vi "GFITS_API.vi"(0 "modpath":path, 7 "Cmd":string, 11 "error in":errorcluster) -> (4 "ImmedReplyString":string, 15 "error out":errorcluster)   [LabVIEW 2016]
uses:
  DBSHAND/private/vis/DatabaseHand_Element_Set(string).vi
  DBSHAND/private/vis/DatabaseHand_Element_Set(bool).vi
  DBSHAND/private/vis/DatabaseHand_Element_Get(U32).vi
  DBSHAND/private/vis/DatabaseHand_Element_Get(string).vi
  DBSHAND/private/vis/DatabaseHand_Element_Get(bool).vi
  DBSHAND/private/vis/DatabaseHand_Element_Get(I32).vi
  private/vis/GFITS_Gbls.vi
panel:
  out "origautonum":bool
  in  "cmd struct":T1
  out "auxhdr":path
  out "caller path":path
  in  "Module vi name":string="GFITS_Main.vi"
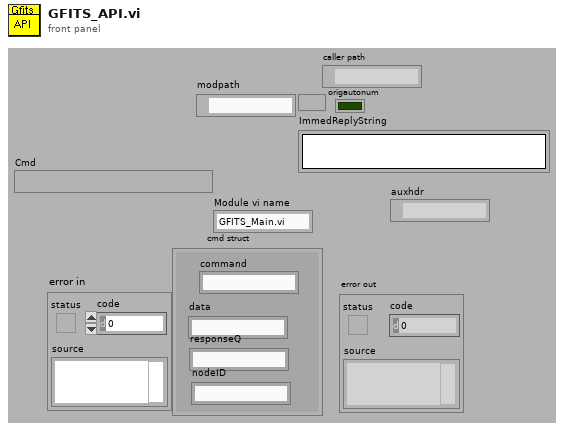
[diagram p1: front panel]
types:
  T1 = cluster{"command":string, "data":string, "responseQ":string, "nodeID":string}
  T2 = typedef "DatabaseHand_RefNum.ctl" = refnum<vi>
  T3 = cluster{"name":string, "Path":path, "bitpix":i8, "naxis":u8, "naxes":u32[], "datatype":u16, "multiple extensions":bool, "hdutype":u16, "writeToDisk":bool, "num_of_ext":u8, "file ref":i32, "createnewimage":bool}
  T4 = cluster{"Name":string, "size (bytes)":u32, "pointer":u32, "Lock":bool}
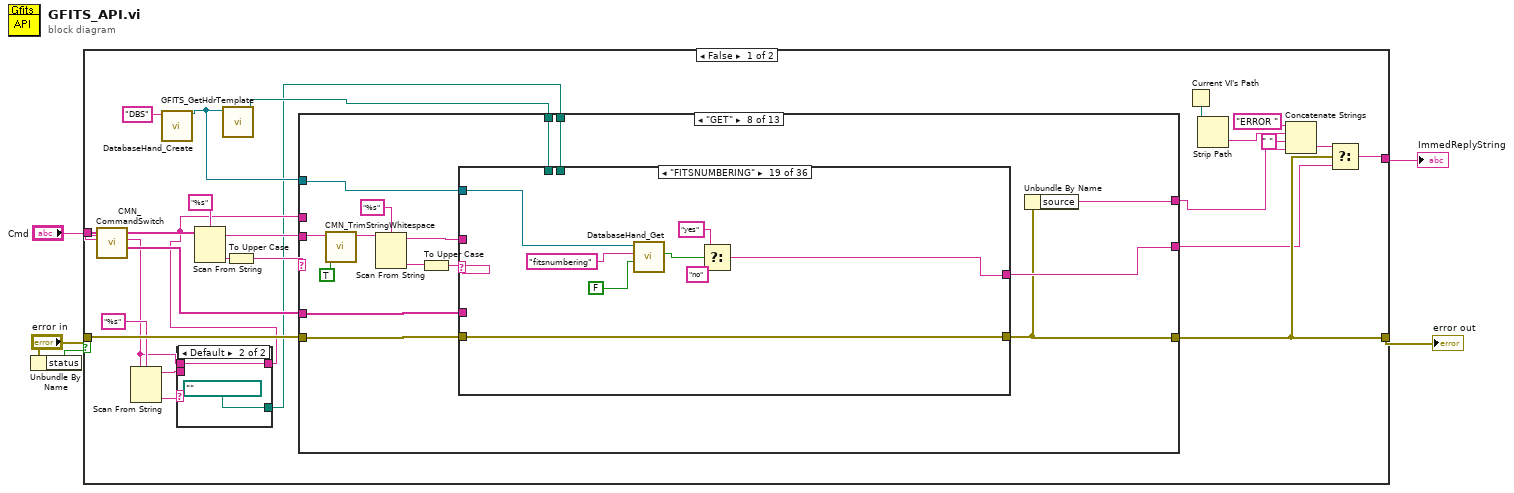
[diagram p0: block diagram]
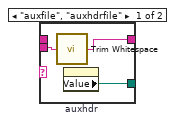
[diagram p2: hidden frame]
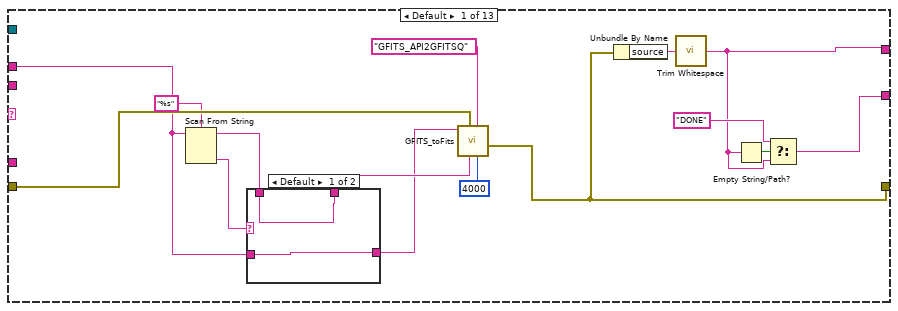
[diagram p3: hidden frame]
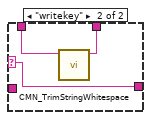
[diagram p4: hidden frame]
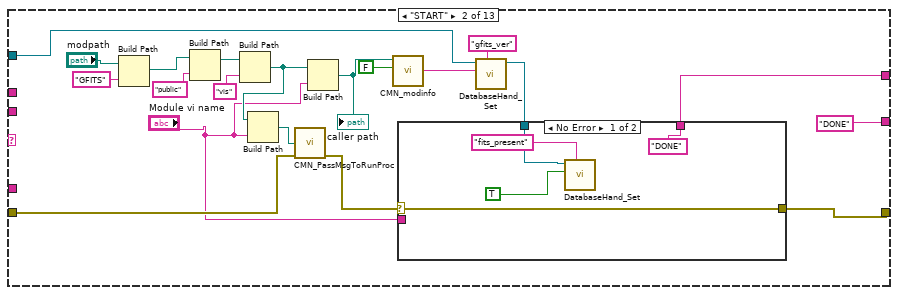
[diagram p5: hidden frame]
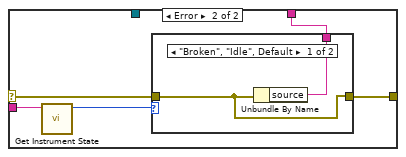
[diagram p6: hidden frame]
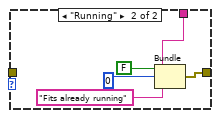
[diagram p7: hidden frame]
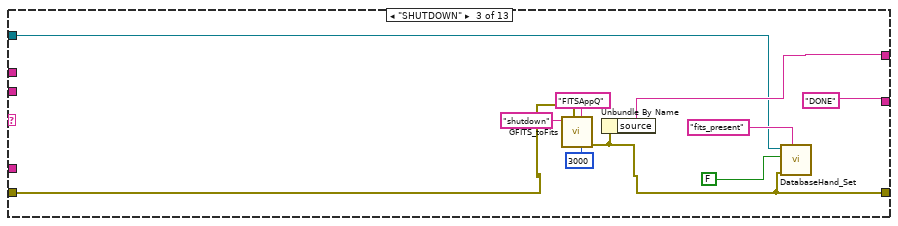
[diagram p8: hidden frame]
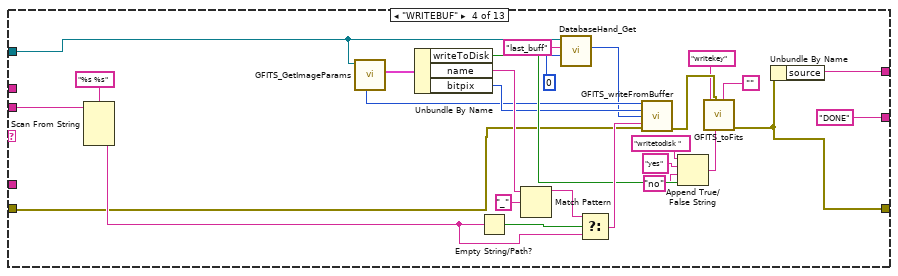
[diagram p9: hidden frame]
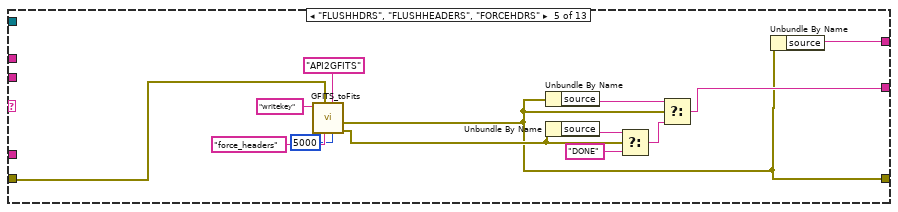
[diagram p10: hidden frame]
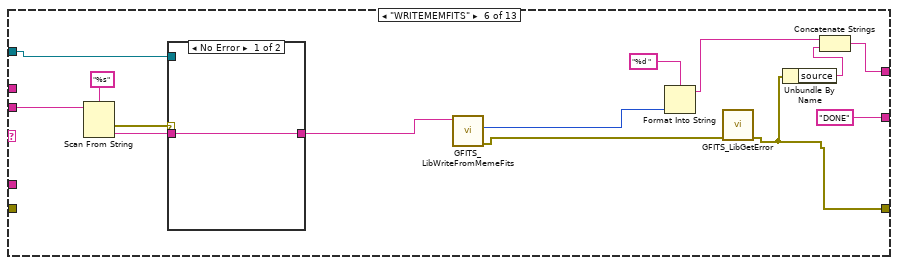
[diagram p11: hidden frame]
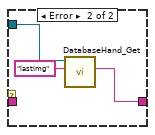
[diagram p12: hidden frame]
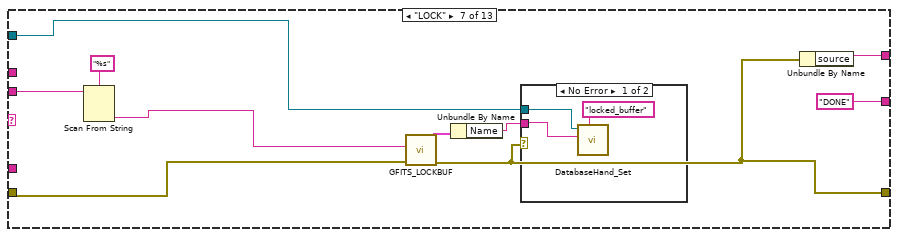
[diagram p13: hidden frame]
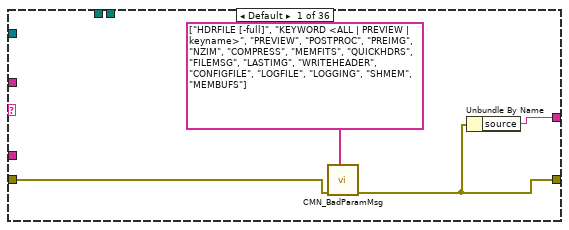
[diagram p15: hidden frame]
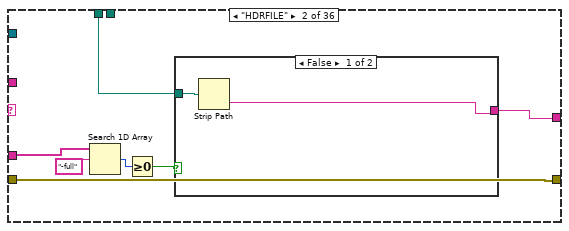
[diagram p16: hidden frame]
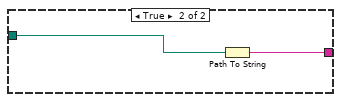
[diagram p17: hidden frame]
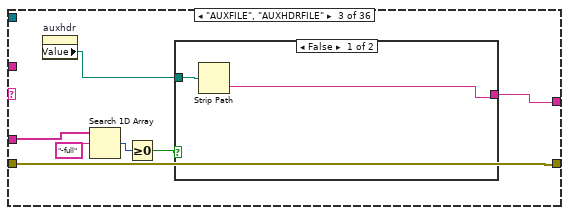
[diagram p18: hidden frame]
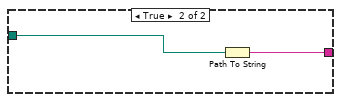
[diagram p19: hidden frame]
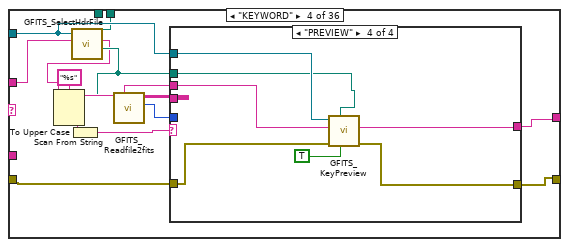
[diagram p20: hidden frame]
diagram:
  n1 = Unbundle By Name("error in") -> ("status"=w3:bool)
  n2 = case shown="False" w3 {
    tunnel: "error in" -> [w30 w1388]
    tunnel: [w23 w1388] -> w1
    tunnel: [w22 ""] -> w5
    tunnel: "Cmd" -> [w19 _]
    frame False {
      n3 = call "CMN_CommandSwitch.vi"("command in"=w19) -> ("swhitches"=w18:string[], "command out"=w9:string)  [unwired: 1 in, 8 out]
      n4 = Scan From String(format string="%s", input string=w9) -> (remaining string=w7:string, output 1=w10:string)  [unwired: 2 in, 3 out]
      n5 = call "DatabaseHand_Create.vi"("Name"="DBS") -> ("Database RefNum out"=w15:T2)  [unwired: 1 in, 9 out]
      n6 = case shown="Default" w10 {
        tunnel: w9 -> [_ w35]
        tunnel: [w32 w35] -> w8
        tunnel: w7 -> [w33 _]
        tunnel: [w31 path "" ("auxhdr")] -> w6
        frame "auxfile", "auxhdrfile" {
          n7 = call <vilib>:"Trim Whitespace.vi"("string"=w33) -> ("trimmed string"=w32:string)  [unwired: 1 in]
          n8 = property on="auxhdr" class="Path"() -> ("Value"=w31:path)  [unwired: 2 in, 2 out]
        }
        frame Default {
        }
      }
      n9 = Scan From String(format string="%s" ("Format String"), input string=w8) -> (remaining string=w20:string, output 1=w29:string)  [unwired: 2 in, 3 out]
      n10 = call "GFITS_GetHdrTemplate.vi"("Database RefNum"=w15) -> ("path"=w16:path)  [unwired: 10 out]
      n11 = To Upper Case(1:w29) -> (0:w14:string)
      n12 = case shown="\"GET\"" w14 {
        selector: w14 -> [_ _ _ _ _ _ _ _ _ _ _ _ w1386]
        tunnel: w30 -> [w49 w58 w100 w110 w129 _ w166 w180 w501 w1241 w1366 w1370 w1385]
        tunnel: [w48 w74 w93 w120 w130 w145 w163 w179 w500 w1240 w1365 w1370 w1384] -> w23
        tunnel: [w42 w61 w99 w125 w141 w142 w164 w185 w506 w1245 w1367 w1371 w1383] -> w13
        tunnel: [w41 "DONE" "DONE" "DONE" w131 "DONE" "DONE" w181 w502 w1242 w1367 w1371 w1383] -> w21
        tunnel: w20 -> [_ _ _ w128 _ w155 w169 w187 w508 w1247 _ w1369 _]
        tunnel: w18 -> [_ _ _ _ _ _ _ w178 w498 _ w1364 _ _]
        tunnel: w16 -> [_ _ _ _ _ _ _ w177 w497 w1236 _ _ _]
        tunnel: w15 -> [_ w62 w92 w102 _ w149 w160 w175 w496 w1238 _ _ _]
        tunnel: w8 -> [w36 _ _ _ _ _ _ _ _ _ _ _ _]
        tunnel: w6 -> [_ _ _ _ _ _ _ w173 w494 w1232 _ _ _]
        frame Default {
          n13 = Scan From String(format string="%s", input string=w36) -> (remaining string=w39:string, output 1=w40:string)  [unwired: 2 in, 3 out]
          n14 = case shown="Default" w40 {
            selector: w40 -> [_ w53]
            tunnel: w39 -> [w51 w55]
            tunnel: [w51 w54] -> w38
            tunnel: [w52 w53] -> w37
            tunnel: w36 -> [w52 _]
            frame Default {
            }
            frame "writekey" {
              n15 = call "CMN_TrimStringWhitespace.vi"("string"=w55) -> ("trimmed string"=w54:string)  [unwired: 1 in, 8 out]
            }
          }
          n16 = call "GFITS_toFits.vi"("ms timeout (-1)"=4000, "response Q"="GFITS_API2GFITSQ", "key"=w38, "error in (no error)"=w49, "command"=w37) -> ("response"=w48:errorcluster)  [unwired: 4 in, 2 out]
          n17 = Unbundle By Name(w48) -> ("source"=w47:string)
          n18 = call <vilib>:"Trim Whitespace.vi"("string"=w47) -> ("trimmed string"=w42:string)  [unwired: 1 in]
          n19 = Empty String/Path?(string/path=w42) -> (empty?=w44:bool)
          n20 = Select(t="DONE", s=w44, f=w42) -> (s? t:f=w41:string)
        }
        frame "START" {
          n21 = Build Path(base path="modpath", name or relative path="GFITS") -> (appended path=w69:path)
          n22 = Build Path(base path=w69, name or relative path="public") -> (appended path=w71:path)
          n23 = Build Path(base path=w71, name or relative path="vis") -> (appended path=w60:path)
          n24 = Build Path(base path=w60, name or relative path="Module vi name") -> (appended path=w59:path)
          n25 = call "CMN_PassMsgToRunProc.vi"("VItoRun"=w59, "error in (no error)"=w58) -> ("error out"=w75:errorcluster)  [unwired: 1 in, 12 out]
          n26 = Build Path(base path=w60, name or relative path="Module vi name") -> (appended path=w66:path)
          "caller path" <- w66
          n27 = call "CMN_modinfo.vi"("full"=FALSE, "caller path"=w66) -> ("INFO"=w63:string)  [unwired: 1 in, 8 out]
          n28 = call-poly "DatabaseHand_Set.vi"("name"="gfits_ver", "value"=w63, "Database RefNum in"=w62) -> ("Database RefNum out"=w56:T2)  [unwired: 5 in, 3 out]
          n29 = case shown="No Error" w75 {
            selector: w75 -> [w80 w85]
            tunnel: [w80 w81] -> w74
            tunnel: ["DONE" ("source") w84] -> w61
            tunnel: "Module vi name" -> [_ w83]
            tunnel: w56 -> [w78 _]
            frame No Error {
              n30 = call-poly "DatabaseHand_Set.vi"("name"="fits_present", "value"=TRUE ("full"), "Database RefNum in"=w78) -> ()  [unwired: 5 in, 4 out]
            }
            frame Error {
              n31 = call <vilib>:"Get Instrument State.vi"("VI name"=w83) -> ("vi state"=w82:enum32{"Broken", "Idle", "Running"})  [unwired: 1 in, 9 out]
              n32 = case shown="\"Broken\", \"Idle\", Default" w82 {
                tunnel: w85 -> [w86 _]
                tunnel: [w87 w88] -> w84
                tunnel: [w86 w91] -> w81
                frame "Broken", "Idle", Default {
                  n33 = Unbundle By Name(w86) -> ("source"=w87:string)
                }
                frame "Running" {
                  w88 = "Fits already running"
                  n34 = Bundle(FALSE, 0, w88) -> (w91:errorcluster)  [unwired: 1 out]
                }
              }
            }
          }
        }
        frame "SHUTDOWN" {
          n35 = call "GFITS_toFits.vi"("ms timeout (-1)"=3000, "response Q"="FITSAppQ", "error in (no error)"=w100, "command"="shutdown" ("Command")) -> ("error out"=w93:errorcluster)  [unwired: 5 in, 2 out]
          n36 = Unbundle By Name(w93) -> ("source"=w99:string)
          n37 = call-poly "DatabaseHand_Set.vi"("name"="fits_present", "error in (no error)"=w93, "value"=FALSE ("full"), "Database RefNum in"=w92) -> ()  [unwired: 4 in, 4 out]
        }
        frame "WRITEBUF" {
          n38 = Scan From String(format string="%s %s" ("Format String"), input string=w128) -> (output 2=w123:string)  [unwired: 2 in, 6 out]
          n39 = call "GFITS_GetImageParams.vi"("Database RefNum"=w102) -> ("imageStruct"=w107:T3, "totele"=w106:u32)  [unwired: 1 in, 8 out]
          n40 = Unbundle By Name(w107) -> ("writeToDisk"=w118:bool, "name"=w113:string, "bitpix"=w109:i8)
          n41 = Empty String/Path?(string/path=w123) -> (empty?=w124:bool)
          n42 = Match Pattern(string=w113, regular expression="_") -> (before substring=w111:string)  [unwired: 4 out]
          n43 = call-poly "DatabaseHand_Get.vi"("default value"=u32 0 ("last_buff"), "name"="last_buff", "Database RefNum in"=w102) -> ("value"=w103:u32)  [unwired: 2 in, 6 out]
          n44 = Select(t=w111, s=w124, f=w123) -> (s? t:f=w122:string)
          n45 = call "GFITS_writeFromBuffer.vi"("total pixels"=w106, "bpp"=w109, "buffer pointer"=w103, "name"=w122, "error in (no error)"=w110) -> ("error out"=w121:errorcluster)  [unwired: 2 in, 8 out]
          n46 = Append True/False String(1:w118, 2:"no" ("false string"), 3:"yes" ("true string"), 4:"writetodisk " ("string (\"\")")) -> (0:w114:string)
          n47 = call "GFITS_toFits.vi"("response Q"="", "key"=w114, "error in (no error)"=w121, "command"="writekey") -> ("error out"=w120:errorcluster)  [unwired: 5 in, 2 out]
          n48 = Unbundle By Name(w120) -> ("source"=w125:string)
        }
        frame "FLUSHHDRS", "FLUSHHEADERS", "FORCEHDRS" {
          n49 = call "GFITS_toFits.vi"("ms timeout (-1)"=5000, "response Q"="API2GFITS", "key"="force_headers", "error in (no error)"=w129, "command"="writekey") -> ("error out"=w132:errorcluster, "response"=w130:errorcluster)  [unwired: 4 in, 1 out]
          n50 = Unbundle By Name(w130) -> ("source"=w136:string)
          n51 = Unbundle By Name(w132) -> ("source"=w135:string)
          n52 = Select(t=w135, s=w132, f="DONE") -> (s? t:f=w134:string)
          n53 = Select(t=w136, s=w130, f=w134) -> (s? t:f=w131:string)
          n54 = Unbundle By Name(w130) -> ("source"=w141:string)
        }
        frame "WRITEMEMFITS" {
          n55 = Scan From String(format string="%s" ("Format String"), input string=w155) -> (error out=w152:errorcluster, output 1=w151:string)  [unwired: 2 in, 3 out]
          n56 = case shown="No Error" w152 {
            tunnel: w151 -> [w156 _]
            tunnel: [w156 w157] -> w150
            tunnel: w149 -> [_ w159]
            frame No Error {
            }
            frame Error {
              n57 = call-poly "DatabaseHand_Get.vi"("name"="lastimg", "Database RefNum in"=w159) -> ("value"=w157:string)  [unwired: 3 in, 6 out]
            }
          }
          n58 = call "GFITS_LibWriteFromMemeFits.vi"("imname"=w150) -> ("error out"=w146:errorcluster, "return value"=w148:i32)  [unwired: 1 in, 8 out]
          n59 = Format Into String(format string="%d ", w148) -> (resulting string=w144:string)  [unwired: 2 in, 1 out]
          n60 = call "GFITS_LibGetError.vi"("error in (no error)"=w146) -> ("error out"=w145:errorcluster)  [unwired: 10 out]
          n61 = Unbundle By Name(w145) -> ("source"=w143:string)
          n62 = Concatenate Strings(w144, w143) -> (w142:string)
        }
        frame "LOCK" {
          n63 = Scan From String(format string="%s" ("Format String"), input string=w169) -> (output 1=w165:string)  [unwired: 2 in, 4 out]
          n64 = call "GFITS_LOCKBUF.vi"("error in"=w166, "bufname"=w165) -> ("error out"=w163:errorcluster, "locked buffer"=w162:T4)  [unwired: 8 out]
          n65 = Unbundle By Name(w162) -> ("Name"=w161:string)
          n66 = case shown="No Error" w163 {
            tunnel: w161 -> [w170 _]
            tunnel: w160 -> [w172 _]
            frame No Error {
              n67 = call-poly "DatabaseHand_Set.vi"("name"="locked_buffer", "value"=w170, "Database RefNum in"=w172) -> ()  [unwired: 5 in, 4 out]
            }
            frame Error {
            }
          }
          n68 = Unbundle By Name(w163) -> ("source"=w164:string)
        }
        frame "GET" {
          n69 = call "CMN_TrimStringWhitespace.vi"("Both Ends?(T)"=TRUE, "string"=w187) -> ("trimmed string"=w184:string)  [unwired: 8 out]
          n70 = Scan From String(format string="%s" ("Format String"), input string=w184) -> (remaining string=w176:string, output 1=w183:string)  [unwired: 2 in, 3 out]
          n71 = To Upper Case(1:w183) -> (0:w174:string)
          n72 = case shown="\"FITSNUMBERING\"" w174 {
            tunnel: [w188 w198 w209 w221 w265 w268 w273 w279 w285 w292 w299 w307 w315 w323 w331 w339 w345 w349 w357 w368 w376 w384 w389 w398 w405 w412 w419 w426 w433 w438 w448 w450 w463 w471 w477 w480] -> w181
            tunnel: w180 -> [w190 w197 w208 w222 w267 w271 w276 w282 w288 w295 w302 w310 w318 w326 w334 w342 w344 w355 w363 w371 w379 w387 w395 w401 w408 w415 w422 w429 w436 w440 w445 w456 w467 w473 w479 w487]
            tunnel: [w189 w197 w208 w220 w266 w271 w275 w281 w287 w294 w301 w309 w317 w325 w333 w341 w344 w355 w363 w370 w378 w386 w395 w400 w407 w414 w421 w428 w435 w439 w445 w456 w467 w473 w479 w486] -> w179
            tunnel: w178 -> [_ w196 w207 _ _ _ _ _ _ _ _ _ _ _ _ _ _ _ _ _ _ _ _ _ _ _ _ _ _ _ _ _ _ _ _ _]
            tunnel: w177 -> [_ w192 _ _ _ _ _ _ _ _ _ _ _ _ _ _ _ _ _ _ _ _ _ _ _ _ _ _ _ _ _ _ _ _ _ _]
            tunnel: w176 -> [_ _ _ w214 w263 w269 _ _ _ _ _ _ _ _ _ _ _ _ _ _ _ _ _ _ _ _ _ _ _ _ _ w451 _ _ _ _]
            tunnel: w175 -> [_ _ _ w218 w264 w270 _ _ _ _ _ _ _ _ _ _ w348 w356 w364 _ _ _ w394 _ _ _ _ _ _ _ w449 w455 _ _ _ _]
            tunnel: w173 -> [_ _ _ w217 w260 _ _ _ _ _ _ _ _ _ _ _ _ _ _ _ _ _ _ _ _ _ _ _ _ _ _ _ _ _ _ _]
            frame Default {
              n73 = call "CMN_BadParamMsg.vi"("valid params"=string[] ["HDRFILE [-full]", "KEYWORD <ALL | PREVIEW | keyname>", "PREVIEW", "POSTPROC", "PREIMG", "NZIM", "COMPRESS", "MEMFITS", "QUICKHDRS", "FILEMSG", "LASTIMG", "WRITEHEADER", "CONFIGFILE", "LOGFILE", "LOGGING", "SHMEM", "MEMBUFS"], "error in (no error)"=w190) -> ("error out"=w189:errorcluster)  [unwired: 2 in, 7 out]
              n74 = Unbundle By Name(w189) -> ("source"=w188:string)
            }
            frame "HDRFILE" {
              n75 = Search 1D Array(1D array=w196, element="-full") -> (index of element=w194:i32)  [unwired: 1 out]
              n76 = Greater Or Equal To 0?(x=w194) -> (x >= 0?=w193:bool)
              n77 = case shown="False" w193 {
                tunnel: [w199 w202] -> w198
                tunnel: w192 -> [w200 w201]
                frame False {
                  n78 = Strip Path(path=w200) -> (name=w199:string)  [unwired: 1 out]
                }
                frame True {
                  n79 = Path To String(path=w201) -> (string=w202:string)
                }
              }
            }
            frame "AUXFILE", "AUXHDRFILE" {
              n80 = property on="auxhdr" class="Path"() -> ("Value"=w203:path)  [unwired: 2 in, 2 out]
              n81 = Search 1D Array(1D array=w207, element="-full") -> (index of element=w205:i32)  [unwired: 1 out]
              n82 = Greater Or Equal To 0?(x=w205) -> (x >= 0?=w204:bool)
              n83 = case shown="False" w204 {
                tunnel: [w210 w213] -> w209
                tunnel: w203 -> [w211 w212]
                frame False {
                  n84 = Strip Path(path=w211) -> (name=w210:string)  [unwired: 1 out]
                }
                frame True {
                  n85 = Path To String(path=w212) -> (string=w213:string)
                }
              }
            }
            frame "KEYWORD" {
              n86 = call "GFITS_SelectHdrFile.vi"("auxhdr"=w217, "line in"=w214, "Database RefNum"=w218) -> ("path out"=w216:path, "line out"=w215:string)  [unwired: 7 out]
              n87 = Scan From String(format string="%s" ("Format String"), input string=w215) -> (remaining string=w219:string, output 1=w224:string)  [unwired: 2 in, 3 out]
              n88 = To Upper Case(1:w224) -> (0:w223:string)
              n89 = call "GFITS_Readfile2fits.vi"("file"=w216) -> ("number of after keywords"=w225:i32, "after Keywords"=w226:string[][])  [unwired: 1 in, 8 out]
              n90 = case shown="\"PREVIEW\"" w223 {
                selector: w223 -> [_ w240 _ _]
                tunnel: w226 -> [_ w242 w250 _]
                tunnel: w216 -> [_ _ w249 w253]
                tunnel: w225 -> [_ _ _ _]
                tunnel: [w229 w235 w246 w256] -> w221
                tunnel: w222 -> [w232 w233 w248 w258]
                tunnel: [w231 w233 w247 w257] -> w220
                tunnel: w218 -> [_ _ _ w255]
                tunnel: w219 -> [_ _ _ w254]
                frame "", " " {
                  w229 = " nothing to get"
                  n91 = Bundle By Name(cluster=w232, "source"=w229, "code"=-22, "status"=FALSE) -> (w231:errorcluster)
                }
                frame Default {
                  w239 = 0 ("Index")
                  n92 = Build Array(w242) -> (w241:string[][][])
                  n93 = call "GFITS_FindKeywordFromArray.vi"("Keyword"=w240, "Keywords"=w241) -> ("values"=w237:string[][], "indexes"=w238:i16[])  [unwired: 8 out]
                  n94 = Index Array(array=w238, index=w239) -> (element=w236:i16)
                  n95 = Index Array(array=w237, index (row)=w239) -> (element=w234:string[])  [unwired: 1 in]
                  n96 = case shown="Default" w236 {
                    tunnel: ["NOT FOUND" w244] -> w235
                    tunnel: w234 -> [_ w245]
                    frame -1 {
                    }
                    frame Default {
                      n97 = call "CMN_Arr2Str.vi"("Array in"=w245) -> ("string out"=w244:string)  [unwired: 10 out]
                    }
                  }
                }
                frame "ALL" {
                  n98 = call "GFITS_Fits2File.vi"("write to file?"=FALSE, "error in (no error)"=w248, "Keywords"=w250, "filename"=w249) -> ("error out"=w247:errorcluster, "string out"=w246:string)  [unwired: 1 in, 5 out]
                }
                frame "PREVIEW" {
                  n99 = call "GFITS_KeyPreview.vi"("nd queue"=TRUE, "template path"=w253, "error in (no error)"=w258, "args"=w254, "Database RefNum in"=w255) -> ("error out"=w257:errorcluster, "preview"=w256:string)  [unwired: 5 out]
                }
              }
            }
            frame "PREVIEW" {
              n100 = call "GFITS_SelectHdrFile.vi"("auxhdr"=w260, "line in"=w263, "Database RefNum"=w264) -> ("path out"=w261:path, "line out"=w262:string)  [unwired: 7 out]
              n101 = call "GFITS_KeyPreview.vi"("nd queue"=TRUE, "template path"=w261, "error in (no error)"=w267, "args"=w262, "Database RefNum in"=w264) -> ("error out"=w266:errorcluster, "preview"=w265:string)  [unwired: 5 out]
            }
            frame "GEOMPREVIEW", "GEOMUPDATE" {
              n102 = call "GFITS_GeomKeyPreview.vi"("args"=w269, "Database RefNum in"=w270) -> ("preview"=w268:string)  [unwired: 1 in, 8 out]
            }
            frame "CONFIGFILE" {
              n103 = call "GFITS_toFits.vi"("response Q"="API2GFITS", "error in (no error)"=w276, "command"="GET CONFIGFILE") -> ("error out"=w275:errorcluster, "response"=w274:errorcluster)  [unwired: 6 in, 1 out]
              n104 = Unbundle By Name(w274) -> ("source"=w273:string)
            }
            frame "LOGFILE" {
              n105 = call "GFITS_toFits.vi"("response Q"="API2GFITS", "error in (no error)"=w282, "command"="GET LOGFILE") -> ("error out"=w281:errorcluster, "response"=w280:errorcluster)  [unwired: 6 in, 1 out]
              n106 = Unbundle By Name(w280) -> ("source"=w279:string)
            }
            frame "LOGGING" {
              n107 = call "GFITS_toFits.vi"("response Q"="API2GFITS", "error in (no error)"=w288, "command"="GET LOGGING") -> ("error out"=w287:errorcluster, "response"=w286:errorcluster)  [unwired: 6 in, 1 out]
              n108 = Unbundle By Name(w286) -> ("source"=w285:string)
            }
            frame "MEMBUF" {
              n109 = call "GFITS_toFits.vi"("response Q"="API2GFITS", "key"="get_membufptr", "error in (no error)"=w295, "command"="writekey") -> ("error out"=w294:errorcluster, "response"=w293:errorcluster)  [unwired: 5 in, 1 out]
              n110 = Unbundle By Name(w293) -> ("source"=w292:string)
            }
            frame "EXTENSIONSMAP", "EXTMAP", "MAPEXTENSIONS" {
              n111 = call "GFITS_toFits.vi"("response Q"="API2GFITS", "key"="get_extensionsmap", "error in (no error)"=w302, "command"="writekey") -> ("error out"=w301:errorcluster, "response"=w300:errorcluster)  [unwired: 5 in, 1 out]
              n112 = Unbundle By Name(w300) -> ("source"=w299:string)
            }
            frame "MEMFITS" {
              n113 = call "GFITS_toFits.vi"("ms timeout (-1)"=5000, "response Q"="API2GFITS", "key"="get_memfits", "error in (no error)"=w310, "command"="writekey") -> ("error out"=w309:errorcluster, "response"=w308:errorcluster)  [unwired: 4 in, 1 out]
              n114 = Unbundle By Name(w308) -> ("source"=w307:string)
            }
            frame "MEMHDRS" {
              n115 = call "GFITS_toFits.vi"("ms timeout (-1)"=5000, "response Q"="API2GFITS", "key"="get_memhdrs", "error in (no error)"=w318, "command"="writekey") -> ("error out"=w317:errorcluster, "response"=w316:errorcluster)  [unwired: 4 in, 1 out]
              n116 = Unbundle By Name(w316) -> ("source"=w315:string)
            }
            frame "POSTPROC" {
              n117 = call "GFITS_toFits.vi"("ms timeout (-1)"=5000, "response Q"="API2GFITS", "key"="get_postproc", "error in (no error)"=w326, "command"="writekey") -> ("error out"=w325:errorcluster, "response"=w324:errorcluster)  [unwired: 4 in, 1 out]
              n118 = Unbundle By Name(w324) -> ("source"=w323:string)
            }
            frame "PREIMAGE", "PREIMAGESCRIPT", "PREIMG" {
              n119 = call "GFITS_toFits.vi"("ms timeout (-1)"=5000, "response Q"="API2GFITS", "key"="get_preimg", "error in (no error)"=w334, "command"="writekey") -> ("error out"=w333:errorcluster, "response"=w332:errorcluster)  [unwired: 4 in, 1 out]
              n120 = Unbundle By Name(w332) -> ("source"=w331:string)
            }
            frame "TESTDIR", "TMPDIR" {
              n121 = call "GFITS_toFits.vi"("ms timeout (-1)"=5000, "response Q"="API2GFITS", "key"="get_testdir", "error in (no error)"=w342, "command"="writekey") -> ("error out"=w341:errorcluster, "response"=w340:errorcluster)  [unwired: 4 in, 1 out]
              n122 = Unbundle By Name(w340) -> ("source"=w339:string)
            }
            frame "IGNORENAME" {
              n123 = call-poly "DatabaseHand_Get.vi"("default value"="none", "name"="ignorename", "Database RefNum in"=w348) -> ("value"=w345:string)  [unwired: 2 in, 6 out]
            }
            frame "FITSOVERRIDE", "OVERRIDE" {
              n124 = call-poly "DatabaseHand_Get.vi"("default value"=FALSE, "name"="fitsoverride", "Database RefNum in"=w356) -> ("value"=w352:bool)  [unwired: 2 in, 6 out]
              n125 = Select(t="yes", s=w352, f="no") -> (s? t:f=w349:string)
            }
            frame "FITSNUMBERING" {
              n126 = call-poly "DatabaseHand_Get.vi"("default value"=FALSE, "name"="fitsnumbering", "Database RefNum in"=w364) -> ("value"=w360:bool)  [unwired: 2 in, 6 out]
              n127 = Select(t="yes", s=w360, f="no") -> (s? t:f=w357:string)
            }
            frame "TESTFNAME" {
              n128 = call "GFITS_toFits.vi"("ms timeout (-1)"=5000, "response Q"="API2GFITS", "key"="get_testfname", "error in (no error)"=w371, "command"="writekey") -> ("error out"=w370:errorcluster, "response"=w369:errorcluster)  [unwired: 4 in, 1 out]
              n129 = Unbundle By Name(w369) -> ("source"=w368:string)
            }
            frame "TESTMODE", "TMPMODE" {
              n130 = call "GFITS_toFits.vi"("ms timeout (-1)"=5000, "response Q"="API2GFITS", "key"="get_testmode", "error in (no error)"=w379, "command"="writekey") -> ("error out"=w378:errorcluster, "response"=w377:errorcluster)  [unwired: 4 in, 1 out]
              n131 = Unbundle By Name(w377) -> ("source"=w376:string)
            }
            frame "POSTIMAGE", "POSTIMAGESCRIPT", "POSTIMG" {
              n132 = call "GFITS_toFits.vi"("ms timeout (-1)"=5000, "response Q"="API2GFITS", "key"="get_postimg", "error in (no error)"=w387, "command"="writekey") -> ("error out"=w386:errorcluster, "response"=w385:errorcluster)  [unwired: 4 in, 1 out]
              n133 = Unbundle By Name(w385) -> ("source"=w384:string)
            }
            frame "DATACUBE", "NZIM", "NZIMAGES", "ZAXIS", "ZIMAGES" {
              n134 = call-poly "DatabaseHand_Get.vi"("default value"=1 ("output 1"), "name"="nzim", "Database RefNum in"=w394) -> ("value"=w391:i32)  [unwired: 2 in, 6 out]
              n135 = Format Into String(format string="%d", w391) -> (resulting string=w389:string)  [unwired: 2 in, 1 out]
            }
            frame "COMPRESS", "COMPRESSION" {
              n136 = call "GFITS_toFits.vi"("response Q"="API2GFITS", "key"="get_compress", "error in (no error)"=w401, "command"="writekey") -> ("error out"=w400:errorcluster, "response"=w399:errorcluster)  [unwired: 5 in, 1 out]
              n137 = Unbundle By Name(w399) -> ("source"=w398:string)
            }
            frame "SHMEM" {
              n138 = call "GFITS_toFits.vi"("response Q"="API2GFITS", "key"="get_shmem", "error in (no error)"=w408, "command"="writekey") -> ("error out"=w407:errorcluster, "response"=w406:errorcluster)  [unwired: 5 in, 1 out]
              n139 = Unbundle By Name(w406) -> ("source"=w405:string)
            }
            frame "QUICKHDRS" {
              n140 = call "GFITS_toFits.vi"("response Q"="API2GFITS", "key"="get_quickhdrs", "error in (no error)"=w415, "command"="writekey") -> ("error out"=w414:errorcluster, "response"=w413:errorcluster)  [unwired: 5 in, 1 out]
              n141 = Unbundle By Name(w413) -> ("source"=w412:string)
            }
            frame "FILEMESSAGE", "FILEMSG" {
              n142 = call "GFITS_toFits.vi"("response Q"="API2GFITS", "key"="get_filemsg", "error in (no error)"=w422, "command"="writekey") -> ("error out"=w421:errorcluster, "response"=w420:errorcluster)  [unwired: 5 in, 1 out]
              n143 = Unbundle By Name(w420) -> ("source"=w419:string)
            }
            frame "ASYNC", "ASYNCMSG", "ASYNCMSGS" {
              n144 = call "GFITS_toFits.vi"("response Q"="API2GFITS", "key"="get_async", "error in (no error)"=w429, "command"="writekey") -> ("error out"=w428:errorcluster, "response"=w427:errorcluster)  [unwired: 5 in, 1 out]
              n145 = Unbundle By Name(w427) -> ("source"=w426:string)
            }
            frame "WRITEHEADER", "WRITEHEADERS" {
              n146 = call "GFITS_toFits.vi"("response Q"="API2GFITS", "key"="get_writeheaders", "error in (no error)"=w436, "command"="writekey") -> ("error out"=w435:errorcluster, "response"=w434:errorcluster)  [unwired: 5 in, 1 out]
              n147 = Unbundle By Name(w434) -> ("source"=w433:string)
            }
            frame "IMAGENUMBERFORMAT", "IMNUMFORMAT", "NUMFORMAT" {
              n148 = call "GFITS_toFits.vi"("response Q"="API2GFITS", "key"="get_imnumformat", "error in (no error)"=w440, "command"="writekey") -> ("error out"=w439:errorcluster, "response"=w443:errorcluster)  [unwired: 5 in, 1 out]
              n149 = Unbundle By Name(w443) -> ("source"=w438:string)
            }
            frame "LASTIMAGE", "LASTIMG" {
              n150 = call-poly "DatabaseHand_Get.vi"("error in (no error)"=w445, "default value"="_none_", "name"="lastimg", "Database RefNum in"=w449) -> ("value"=w448:string)  [unwired: 1 in, 6 out]
            }
            frame "LASTHDR", "LASTHDRS" {
              n151 = call-poly "DatabaseHand_Get.vi"("default value"=FALSE, "name"="memhdrs", "Database RefNum in"=w455) -> ("value"=w452:bool)  [unwired: 2 in, 6 out]
              n152 = case shown="True" w452 {
                tunnel: w451 -> [_ w459]
                tunnel: ["No record.  To start recording please set \"memhdrs\" to \"on\"" ("hdrs") w458] -> w450
                frame False {
                }
                frame True {
                  n153 = call "GFITS_GetLastHdrs.vi"("ext"=w459) -> ("hdrs"=w458:string)  [unwired: 10 out]
                }
              }
            }
            frame "HDRPREALLOC", "KEYPREALLOC" {
              n154 = call "GFITS_VAR_preallocHdrs.vi"("action"=enum16{"read", "write"}."read") -> ("nkeys out"=w462:i32)  [unwired: 1 in, 13 out]
              n155 = Format Into String(format string="%d", w462) -> (resulting string=w461:string)  [unwired: 2 in, 1 out]
              n156 = Greater Or Equal To 0?(x=w462) -> (x >= 0?=w465:bool)
              n157 = Select(t=w461, s=w465, f="auto") -> (s? t:f=w463:string)
            }
            frame "HDRMODE", "KEYMODE" {
              n158 = call "GFITS_VAR_staticHdrs.vi"("action"=enum16{"read", "write"}."read") -> ("static out"=w469:bool)  [unwired: 1 in, 13 out]
              n159 = Select(t="static", s=w469, f="dynamic") -> (s? t:f=w471:string)
            }
            frame "GEOMHDRMODE" {
              n160 = call "GFITS_VAR_fstaticGeomHdrs.vi"("action"=enum16{"read", "write"}."read") -> ("static out"=w474:bool)  [unwired: 1 in, 13 out]
              n161 = Select(t="static", s=w474, f="dynamic") -> (s? t:f=w477:string)
            }
            frame "ROI" {
              n162 = call "GFITS_LibGetRoi.vi"("error in (no error)"=w487) -> ("error IO"=w486:errorcluster, "roi?"=w485:bool, "ylen"=w481:u32, "ystart out"=w483:u32, "xlen out"=w482:u32, "xstart out"=w484:u32)  [unwired: 5 out]
              n163 = case shown="False" w485 {
                tunnel: w484 -> [_ w493]
                tunnel: w483 -> [_ w492]
                tunnel: w482 -> [_ w491]
                tunnel: w481 -> [_ w490]
                tunnel: ["none" w489] -> w480
                frame False {
                }
                frame True {
                  n164 = Format Into String(w493, w492, w491, w490) -> (resulting string=w489:string)  [unwired: 3 in, 1 out]
                }
              }
            }
          }
          n165 = Unbundle By Name(w179) -> ("source"=w185:string)
        }
        frame "SET" {
          n166 = call "CMN_TrimStringWhitespace.vi"("Both Ends?(T)"=TRUE, "string"=w508) -> ("trimmed string"=w505:string)  [unwired: 8 out]
          n167 = Scan From String(format string="%s" ("Format String"), input string=w505) -> (remaining string=w499:string, output 1=w504:string)  [unwired: 2 in, 3 out]
          n168 = To Upper Case(1:w504) -> (0:w495:string)
          n169 = case shown="\"FITSNUMBERING\"" w495 {
            tunnel: [w509 w515 w548 "DONE" ("data string") w598 w618 w638 w655 w686 w711 w737 w766 w781 w799 w819 w839 w861 w883 w904 w924 w939 w957 w976 w993 w1010 w1026 w1043 w1050 w1067 w1080 w1106 w1134 w1176 w1205] -> w502
            tunnel: w501 -> [w511 w524 w556 w584 w603 w623 w643 w658 w689 w714 w740 w771 w786 w804 w824 w844 w866 w888 w909 w929 w944 w962 w981 w998 w1015 w1031 w1048 w1060 w1066 w1084 w1109 w1133 w1179 w1200]
            tunnel: [w510 w524 w556 w583 w600 w620 w640 w657 w688 w713 w739 w768 w783 w801 w821 w841 w863 w885 w906 w926 w941 w959 w978 w995 w1012 w1028 w1045 w1051 w1065 w1082 w1107 w1132 w1177 w1206] -> w500
            tunnel: w499 -> [_ w526 w558 w585 w593 w613 w633 w650 w681 w706 w732 w761 w777 w794 w814 w828 w850 w872 w893 w919 w932 w952 w971 w988 w1005 w1021 w1038 w1057 w1064 w1087 w1112 w1138 w1182 w1204]
            tunnel: w498 -> [_ w523 w555 _ _ _ _ _ _ _ _ _ _ _ _ _ _ _ _ _ _ _ _ _ _ _ _ _ _ _ _ _ _ _]
            tunnel: w497 -> [_ w521 w553 _ _ _ _ _ _ _ _ _ _ _ _ _ _ _ _ _ _ _ _ _ _ _ _ _ _ _ _ _ _ _]
            tunnel: w496 -> [_ w514 _ w582 _ _ _ _ w677 _ _ _ _ _ _ _ _ _ _ _ _ _ _ _ _ _ _ _ _ _ _ w1131 _ _]
            tunnel: w494 -> [_ _ _ w581 _ _ _ _ _ _ _ _ _ _ _ _ _ _ _ _ _ _ _ _ _ _ _ _ _ _ _ _ _ _]
            frame Default {
              n170 = call "CMN_BadParamMsg.vi"("valid params"=string[] ["HDRFILE <path>", "KEYWORD <...> (same as KEY ADD)", "AUTOWRITE <on | off>", "MEXT <on | off>", "QUICKHEADERS <on | off>", "MEMFITS <on | off>", "POSTPROC <script | none>", "PREIMG <script | none>", "NBUFS <number_of_buffers>", "COPMPRESSION <algor | none>", "ASYNCMSGS <on | off>", "FILEMSG <format | none>", "HDRVAR <type> <name> <value>", "AUXFILE <path>"], "error in (no error)"=w511) -> ("error out"=w510:errorcluster)  [unwired: 2 in, 7 out]
              n171 = Unbundle By Name(w510) -> ("source"=w509:string)
            }
            frame "HDRFILE" {
              n172 = Search 1D Array(1D array=w523, element="-full") -> (index of element=w520:i32)  [unwired: 1 out]
              n173 = call "CMN_TrimStringWhitespace.vi"("Both Ends?(T)"=TRUE, "string"=w526) -> ("trimmed string"=w518:string)  [unwired: 8 out]
              n174 = Greater Or Equal To 0?(x=w520) -> (x >= 0?=w519:bool)
              n175 = case shown="True" w519 {
                tunnel: w521 -> [w537 _]
                tunnel: w518 -> [w535 w543]
                tunnel: [w534 w538] -> w513
                frame False {
                  n176 = Strip Path(path=w537) -> (stripped path=w536:path)  [unwired: 1 out]
                  n177 = Build Path(base path=w536, name or relative path=w535) -> (appended path=w534:path)
                }
                frame True {
                  n178 = String To Path(string=w543) -> (path=w542:path)
                  n179 = call "CMN_PathParams2Path.vi"("Path In"=w542) -> ("Path out"=w540:path)  [unwired: 2 in, 8 out]
                  n180 = Path To String(path=w540) -> (string=w541:string)
                  n181 = call "CMN_ReplaceName.vi"("name in"=w541) -> ("name out"=w539:string)  [unwired: 1 in, 9 out]
                  n182 = String To Path(string=w539) -> (path=w538:path)
                }
              }
              n183 = call "GFITS_SetHdrTemplate.vi"("path"=w513, "Database RefNum"=w514) -> ()  [unwired: 1 in, 9 out]
              n184 = File/Directory Info(path=w513) -> (directory=w516:bool, error out=w517:errorcluster)  [unwired: 1 in, 5 out]
              n185 = case shown="Error" w517 {
                tunnel: w516 -> [w530 _]
                tunnel: [w527 w532] -> w515
                frame No Error {
                  n186 = Select(t="WRN: is a directory", s=w530, f="DONE" ("data string")) -> (s? t:f=w527:string)
                }
                frame Error {
                  n187 = Concatenate Strings("WARNING: " ("string"), "File does not exists. Set anyway") -> (w532:string)
                }
              }
            }
            frame "AUXFILE", "AUXHDRFILE" {
              n188 = call "CMN_TrimStringWhitespace.vi"("Both Ends?(T)"=TRUE, "string"=w558) -> ("trimmed string"=w546:string)  [unwired: 8 out]
              n189 = Search 1D Array(1D array=w555, element="-full") -> (index of element=w552:i32)  [unwired: 1 out]
              n190 = Scan From String(format string="%s", input string=w546) -> (output 1=w544:string)  [unwired: 2 in, 4 out]
              n191 = Greater Or Equal To 0?(x=w552) -> (x >= 0?=w551:bool)
              n192 = case shown="False" w551 {
                tunnel: w553 -> [w569 _]
                tunnel: w546 -> [w568 w580]
                tunnel: [w567 w575] -> w547
                tunnel: w544 -> [w566 _]
                frame False {
                  n193 = case shown="\"main\", \"none\"" w566 {
                    tunnel: w569 -> [_ w574]
                    tunnel: w568 -> [_ w572]
                    tunnel: [path "" ("auxhdr") w571] -> w567
                    frame "main", "none" {
                    }
                    frame Default {
                      n194 = Strip Path(path=w574) -> (stripped path=w573:path)  [unwired: 1 out]
                      n195 = Build Path(base path=w573, name or relative path=w572) -> (appended path=w571:path)
                    }
                  }
                }
                frame True {
                  n196 = String To Path(string=w580) -> (path=w579:path)
                  n197 = call "CMN_PathParams2Path.vi"("Path In"=w579) -> ("Path out"=w577:path)  [unwired: 2 in, 8 out]
                  n198 = Path To String(path=w577) -> (string=w578:string)
                  n199 = call "CMN_ReplaceName.vi"("name in"=w578) -> ("name out"=w576:string)  [unwired: 1 in, 9 out]
                  n200 = String To Path(string=w576) -> (path=w575:path)
                }
              }
              "auxhdr" <- w547
              n201 = File/Directory Info(path=w547) -> (directory=w549:bool, error out=w550:errorcluster)  [unwired: 1 in, 5 out]
              n202 = case shown="Error" w550 {
                tunnel: w549 -> [w562 _]
                tunnel: [w559 w564] -> w548
                frame No Error {
                  n203 = Select(t="WRN: is a directory", s=w562, f="DONE" ("data string")) -> (s? t:f=w559:string)
                }
                frame Error {
                  n204 = Concatenate Strings("WARNING: " ("string"), "File does not exists. Set anyway") -> (w564:string)
                }
              }
            }
            frame "KEYWORD" {
              n205 = call "GFITS_AddKeyword.vi"("auxhdr"=w581, "Database RefNum"=w582, "error in"=w584, "command in"=w585) -> ("error out"=w583:errorcluster)  [unwired: 7 out]
            }
            frame "AUTOWRIT", "AUTOWRITE" {
              n206 = Scan From String(format string="%s", input string=w593) -> (output 1=w591:string)  [unwired: 2 in, 4 out]
              n207 = To Lower Case(string=w591) -> (all lower case string=w590:string)
              n208 = case shown="\"on\", \"true\", \"yes\"" w590 {
                tunnel: ["no" "yes"] -> w588
                frame Default {
                }
                frame "on", "true", "yes" {
                }
              }
              n209 = Concatenate Strings("writetodisk " ("key"), w588) -> (w587:string)
              n210 = call "GFITS_toFits.vi"("ms timeout (-1)"=4000, "response Q"="API2GFITS", "key"=w587, "error in (no error)"=w603, "command"="writekey") -> ("error out"=w600:errorcluster, "response"=w597:errorcluster)  [unwired: 4 in, 1 out]
              n211 = Unbundle By Name(w600) -> ("source"=w599:string)
              n212 = Unbundle By Name(w597) -> ("source"=w596:string)
              n213 = Select(t=w596, s=w597, f="DONE") -> (s? t:f=w595:string)
              n214 = Select(t=w599, s=w600, f=w595) -> (s? t:f=w598:string)
            }
            frame "FITSOVERRIDE", "OVERRIDE" {
              n215 = Scan From String(format string="%s", input string=w613) -> (output 1=w611:string)  [unwired: 2 in, 4 out]
              n216 = To Lower Case(string=w611) -> (all lower case string=w610:string)
              n217 = case shown="\"1\", \"enable\", \"on\", \"true\", \"yes\"" w610 {
                tunnel: ["no" "yes"] -> w608
                frame Default {
                }
                frame "1", "enable", "on", "true", "yes" {
                }
              }
              n218 = Concatenate Strings("fitsoverride " ("key"), w608) -> (w607:string)
              n219 = call "GFITS_toFits.vi"("ms timeout (-1)"=4000, "response Q"="API2GFITS", "key"=w607, "error in (no error)"=w623, "command"="writekey") -> ("error out"=w620:errorcluster, "response"=w617:errorcluster)  [unwired: 4 in, 1 out]
              n220 = Unbundle By Name(w620) -> ("source"=w619:string)
              n221 = Unbundle By Name(w617) -> ("source"=w616:string)
              n222 = Select(t=w616, s=w617, f="DONE") -> (s? t:f=w615:string)
              n223 = Select(t=w619, s=w620, f=w615) -> (s? t:f=w618:string)
            }
            frame "FITSNUMBERING" {
              n224 = Scan From String(format string="%s", input string=w633) -> (output 1=w631:string)  [unwired: 2 in, 4 out]
              n225 = To Lower Case(string=w631) -> (all lower case string=w630:string)
              n226 = case shown="\"1\", \"enable\", \"on\", \"true\", \"yes\"" w630 {
                tunnel: ["no" "yes"] -> w628
                frame Default {
                }
                frame "1", "enable", "on", "true", "yes" {
                }
              }
              n227 = Concatenate Strings("fitsnumbering " ("key"), w628) -> (w627:string)
              n228 = call "GFITS_toFits.vi"("ms timeout (-1)"=4000, "response Q"="API2GFITS", "key"=w627, "error in (no error)"=w643, "command"="writekey") -> ("error out"=w640:errorcluster, "response"=w637:errorcluster)  [unwired: 4 in, 1 out]
              n229 = Unbundle By Name(w640) -> ("source"=w639:string)
              n230 = Unbundle By Name(w637) -> ("source"=w636:string)
              n231 = Select(t=w636, s=w637, f="DONE") -> (s? t:f=w635:string)
              n232 = Select(t=w639, s=w640, f=w635) -> (s? t:f=w638:string)
            }
            frame "FORCENAME", "MNAME", "NAME", "WRITENEXT" {
              n233 = Scan From String(format string="%s", input string=w650) -> (error out=w648:errorcluster, output 1=w647:string)  [unwired: 2 in, 3 out]
              n234 = case shown="Error" w648 {
                tunnel: w658 -> [w666 w675]
                tunnel: [w663 w672] -> w657
                tunnel: [w662 w671] -> w654
                tunnel: w647 -> [w659 _]
                frame No Error {
                  n235 = Concatenate Strings("forcename " ("key"), w659) -> (w660:string)
                  n236 = call "GFITS_toFits.vi"("ms timeout (-1)"=4000, "response Q"="API2GFITS", "key"=w660, "error in (no error)"=w666, "command"="writekey") -> ("error out"=w663:errorcluster, "response"=w662:errorcluster)  [unwired: 4 in, 1 out]
                }
                frame Error {
                  n237 = Concatenate Strings("forcename " ("key"), "_next_" ("string")) -> (w669:string)
                  n238 = call "GFITS_toFits.vi"("ms timeout (-1)"=4000, "response Q"="API2GFITS", "key"=w669, "error in (no error)"=w675, "command"="writekey") -> ("error out"=w672:errorcluster, "response"=w671:errorcluster)  [unwired: 4 in, 1 out]
                }
              }
              n239 = Unbundle By Name(w657) -> ("source"=w656:string)
              n240 = Unbundle By Name(w654) -> ("source"=w653:string)
              n241 = Select(t=w653, s=w654, f="DONE") -> (s? t:f=w652:string)
              n242 = Select(t=w656, s=w657, f=w652) -> (s? t:f=w655:string)
            }
            frame "IGNORENAME" {
              n243 = Scan From String(format string="%s", input string=w681) -> (error out=w679:errorcluster, output 1=w678:string)  [unwired: 2 in, 3 out]
              n244 = case shown="No Error" w679 {
                tunnel: w689 -> [_ w701]
                tunnel: [w690 w698] -> w688
                tunnel: [w690 w697] -> w685
                tunnel: w678 -> [w691 _]
                tunnel: w677 -> [w693 _]
                frame No Error {
                  n245 = call-poly "DatabaseHand_Set.vi"("name"="ignorename", "value"=w691, "Database RefNum in"=w693) -> ("error out"=w690:errorcluster)  [unwired: 5 in, 3 out]
                }
                frame Error {
                  n246 = Concatenate Strings("forcename " ("key"), "_next_" ("string")) -> (w695:string)
                  n247 = call "GFITS_toFits.vi"("ms timeout (-1)"=4000, "response Q"="API2GFITS", "key"=w695, "error in (no error)"=w701, "command"="writekey") -> ("error out"=w698:errorcluster, "response"=w697:errorcluster)  [unwired: 4 in, 1 out]
                }
              }
              n248 = Unbundle By Name(w688) -> ("source"=w687:string)
              n249 = Unbundle By Name(w685) -> ("source"=w684:string)
              n250 = Select(t=w684, s=w685, f="DONE") -> (s? t:f=w683:string)
              n251 = Select(t=w687, s=w688, f=w683) -> (s? t:f=w686:string)
            }
            frame "TESTDIR", "TMPDIR" {
              n252 = Scan From String(format string="%s", input string=w706) -> (error out=w704:errorcluster, output 1=w703:string)  [unwired: 2 in, 3 out]
              n253 = case shown="No Error" w704 {
                tunnel: w714 -> [w722 w728]
                tunnel: [w719 w724] -> w713
                tunnel: [w718 w724] -> w710
                tunnel: w703 -> [w715 _]
                frame No Error {
                  n254 = Concatenate Strings("testdir " ("key"), w715) -> (w716:string)
                  n255 = call "GFITS_toFits.vi"("ms timeout (-1)"=4000, "response Q"="API2GFITS", "key"=w716, "error in (no error)"=w722, "command"="writekey") -> ("error out"=w719:errorcluster, "response"=w718:errorcluster)  [unwired: 4 in, 1 out]
                }
                frame Error {
                  n256 = Bundle By Name(cluster=w728, "status"=TRUE, "code"=-22, "source"="ERROR bad argument") -> (w724:errorcluster)
                }
              }
              n257 = Unbundle By Name(w713) -> ("source"=w712:string)
              n258 = Unbundle By Name(w710) -> ("source"=w709:string)
              n259 = Select(t=w709, s=w710, f="DONE") -> (s? t:f=w708:string)
              n260 = Select(t=w712, s=w713, f=w708) -> (s? t:f=w711:string)
            }
            frame "TESTBNAME", "TESTNAME" {
              n261 = Scan From String(format string="%s", input string=w732) -> (error out=w730:errorcluster, output 1=w729:string)  [unwired: 2 in, 3 out]
              n262 = case shown="No Error" w730 {
                tunnel: w740 -> [w748 w754]
                tunnel: [w745 w750] -> w739
                tunnel: [w744 w750] -> w736
                tunnel: w729 -> [w741 _]
                frame No Error {
                  n263 = Concatenate Strings("testbname " ("key"), w741) -> (w742:string)
                  n264 = call "GFITS_toFits.vi"("ms timeout (-1)"=4000, "response Q"="API2GFITS", "key"=w742, "error in (no error)"=w748, "command"="writekey") -> ("error out"=w745:errorcluster, "response"=w744:errorcluster)  [unwired: 4 in, 1 out]
                }
                frame Error {
                  n265 = Bundle By Name(cluster=w754, "status"=TRUE, "code"=-22, "source"="ERROR bad argument") -> (w750:errorcluster)
                }
              }
              n266 = Unbundle By Name(w739) -> ("source"=w738:string)
              n267 = Unbundle By Name(w736) -> ("source"=w735:string)
              n268 = Select(t=w735, s=w736, f="DONE") -> (s? t:f=w734:string)
              n269 = Select(t=w738, s=w739, f=w734) -> (s? t:f=w737:string)
            }
            frame "EXTENSIONS", "MEXT" {
              n270 = Scan From String(format string="%s", input string=w761) -> (output 1=w759:string)  [unwired: 2 in, 4 out]
              n271 = To Lower Case(string=w759) -> (all lower case string=w758:string)
              n272 = case shown="\"on\", \"true\", \"yes\"" w758 {
                tunnel: ["no" "yes"] -> w756
                frame Default {
                }
                frame "on", "true", "yes" {
                }
              }
              n273 = Concatenate Strings("mext " ("key"), w756) -> (w755:string)
              n274 = call "GFITS_toFits.vi"("ms timeout (-1)"=4000, "response Q"="API2GFITS", "key"=w755, "error in (no error)"=w771, "command"="writekey") -> ("error out"=w768:errorcluster, "response"=w765:errorcluster)  [unwired: 4 in, 1 out]
              n275 = Unbundle By Name(w768) -> ("source"=w767:string)
              n276 = Unbundle By Name(w765) -> ("source"=w764:string)
              n277 = Select(t=w764, s=w765, f="DONE") -> (s? t:f=w763:string)
              n278 = Select(t=w767, s=w768, f=w763) -> (s? t:f=w766:string)
            }
            frame "EXTENSIONSMAP", "EXTMAP", "MAPEXTENSIONS" {
              n279 = call <vilib>:"Trim Whitespace.vi"("string"=w777) -> ("trimmed string"=w776:string)  [unwired: 1 in]
              n280 = Concatenate Strings("extensionsmap " ("key"), w776) -> (w778:string)
              n281 = call "GFITS_toFits.vi"("ms timeout (-1)"=4000, "response Q"="API2GFITS", "key"=w778, "error in (no error)"=w786, "command"="writekey") -> ("error out"=w783:errorcluster, "response"=w780:errorcluster)  [unwired: 4 in, 1 out]
              n282 = Unbundle By Name(w783) -> ("source"=w782:string)
              n283 = Unbundle By Name(w780) -> ("source"=w775:string)
              n284 = Select(t=w782, s=w783, f=w775) -> (s? t:f=w781:string)
            }
            frame "MEMFITS" {
              n285 = Scan From String(format string="%s", input string=w794) -> (output 1=w792:string)  [unwired: 2 in, 4 out]
              n286 = To Lower Case(string=w792) -> (all lower case string=w791:string)
              n287 = case shown="\"on\", \"true\", \"yes\"" w791 {
                tunnel: ["no" "yes"] -> w789
                frame Default {
                }
                frame "on", "true", "yes" {
                }
              }
              n288 = Concatenate Strings("set_memfits " ("key"), w789) -> (w788:string)
              n289 = call "GFITS_toFits.vi"("ms timeout (-1)"=4000, "response Q"="API2GFITS", "key"=w788, "error in (no error)"=w804, "command"="writekey") -> ("error out"=w801:errorcluster, "response"=w798:errorcluster)  [unwired: 4 in, 1 out]
              n290 = Unbundle By Name(w801) -> ("source"=w800:string)
              n291 = Unbundle By Name(w798) -> ("source"=w797:string)
              n292 = Select(t=w797, s=w798, f="DONE") -> (s? t:f=w796:string)
              n293 = Select(t=w800, s=w801, f=w796) -> (s? t:f=w799:string)
            }
            frame "MEMHDRS" {
              n294 = Scan From String(format string="%s", input string=w814) -> (output 1=w812:string)  [unwired: 2 in, 4 out]
              n295 = To Lower Case(string=w812) -> (all lower case string=w811:string)
              n296 = case shown="\"on\", \"true\", \"yes\"" w811 {
                tunnel: ["no" "yes"] -> w809
                frame Default {
                }
                frame "on", "true", "yes" {
                }
              }
              n297 = Concatenate Strings("set_memhdrs " ("key"), w809) -> (w808:string)
              n298 = call "GFITS_toFits.vi"("ms timeout (-1)"=4000, "response Q"="API2GFITS", "key"=w808, "error in (no error)"=w824, "command"="writekey") -> ("error out"=w821:errorcluster, "response"=w818:errorcluster)  [unwired: 4 in, 1 out]
              n299 = Unbundle By Name(w821) -> ("source"=w820:string)
              n300 = Unbundle By Name(w818) -> ("source"=w817:string)
              n301 = Select(t=w817, s=w818, f="DONE") -> (s? t:f=w816:string)
              n302 = Select(t=w820, s=w821, f=w816) -> (s? t:f=w819:string)
            }
            frame "POSTPROC" {
              n303 = Scan From String(format string="%s", input string=w828) -> (output 1=w833:string)  [unwired: 2 in, 4 out]
              n304 = To Lower Case(string=w833) -> (all lower case string=w832:string)
              n305 = case shown="\"0\", \"false\", \"no\", \"none\", \"off\"" w832 {
                tunnel: [w846 "none"] -> w830
                tunnel: w828 -> [w847 _]
                frame Default {
                  n306 = call <vilib>:"Trim Whitespace.vi"("string"=w847) -> ("trimmed string"=w846:string)  [unwired: 1 in]
                }
                frame "0", "false", "no", "none", "off" {
                }
              }
              n307 = Concatenate Strings("set_postproc " ("key"), w830) -> (w829:string)
              n308 = call "GFITS_toFits.vi"("ms timeout (-1)"=4000, "response Q"="API2GFITS", "key"=w829, "error in (no error)"=w844, "command"="writekey") -> ("error out"=w841:errorcluster, "response"=w838:errorcluster)  [unwired: 4 in, 1 out]
              n309 = Unbundle By Name(w841) -> ("source"=w840:string)
              n310 = Unbundle By Name(w838) -> ("source"=w837:string)
              n311 = Select(t=w837, s=w838, f="DONE") -> (s? t:f=w836:string)
              n312 = Select(t=w840, s=w841, f=w836) -> (s? t:f=w839:string)
            }
            frame "WAITSTAT", "WAITSTATS" {
              n313 = Scan From String(format string="%s", input string=w850) -> (remaining string=w849:string, output 1=w855:string)  [unwired: 2 in, 3 out]
              n314 = To Lower Case(string=w855) -> (all lower case string=w854:string)
              n315 = case shown="Default" w854 {
                tunnel: [w869 "0" "2000"] -> w852
                tunnel: w850 -> [_ _ _]
                tunnel: w849 -> [w868 _ _]
                frame Default {
                  n316 = call <vilib>:"Trim Whitespace.vi"("string"=w868) -> ("trimmed string"=w869:string)  [unwired: 1 in]
                }
                frame "0", "false", "no", "none", "off" {
                }
                frame "on", "true", "yes" {
                }
              }
              n317 = Concatenate Strings("set_waitstats " ("key"), w852) -> (w851:string)
              n318 = call "GFITS_toFits.vi"("ms timeout (-1)"=4000, "response Q"="API2GFITS", "key"=w851, "error in (no error)"=w866, "command"="writekey") -> ("error out"=w863:errorcluster, "response"=w860:errorcluster)  [unwired: 4 in, 1 out]
              n319 = Unbundle By Name(w863) -> ("source"=w862:string)
              n320 = Unbundle By Name(w860) -> ("source"=w859:string)
              n321 = Select(t=w859, s=w860, f="DONE") -> (s? t:f=w858:string)
              n322 = Select(t=w862, s=w863, f=w858) -> (s? t:f=w861:string)
            }
            frame "PREIMAGE", "PREIMG", "PREIMGSCRIPT" {
              n323 = Scan From String(format string="%s", input string=w872) -> (output 1=w877:string)  [unwired: 2 in, 4 out]
              n324 = To Lower Case(string=w877) -> (all lower case string=w876:string)
              n325 = case shown="\"0\", \"false\", \"no\", \"none\", \"off\"" w876 {
                tunnel: [w890 "none"] -> w874
                tunnel: w872 -> [w891 _]
                frame Default {
                  n326 = call <vilib>:"Trim Whitespace.vi"("string"=w891) -> ("trimmed string"=w890:string)  [unwired: 1 in]
                }
                frame "0", "false", "no", "none", "off" {
                }
              }
              n327 = Concatenate Strings("set_preimg " ("key"), w874) -> (w873:string)
              n328 = call "GFITS_toFits.vi"("ms timeout (-1)"=4000, "response Q"="API2GFITS", "key"=w873, "error in (no error)"=w888, "command"="writekey") -> ("error out"=w885:errorcluster, "response"=w882:errorcluster)  [unwired: 4 in, 1 out]
              n329 = Unbundle By Name(w885) -> ("source"=w884:string)
              n330 = Unbundle By Name(w882) -> ("source"=w881:string)
              n331 = Select(t=w881, s=w882, f="DONE") -> (s? t:f=w880:string)
              n332 = Select(t=w884, s=w885, f=w880) -> (s? t:f=w883:string)
            }
            frame "POSTIMAGE", "POSTIMG", "POSTIMGCSRIPT" {
              n333 = Scan From String(format string="%s", input string=w893) -> (output 1=w898:string)  [unwired: 2 in, 4 out]
              n334 = To Lower Case(string=w898) -> (all lower case string=w897:string)
              n335 = case shown="\"0\", \"false\", \"no\", \"none\", \"off\"" w897 {
                tunnel: [w911 "none"] -> w895
                tunnel: w893 -> [w912 _]
                frame Default {
                  n336 = call <vilib>:"Trim Whitespace.vi"("string"=w912) -> ("trimmed string"=w911:string)  [unwired: 1 in]
                }
                frame "0", "false", "no", "none", "off" {
                }
              }
              n337 = Concatenate Strings("set_postimg " ("key"), w895) -> (w894:string)
              n338 = call "GFITS_toFits.vi"("ms timeout (-1)"=4000, "response Q"="API2GFITS", "key"=w894, "error in (no error)"=w909, "command"="writekey") -> ("error out"=w906:errorcluster, "response"=w903:errorcluster)  [unwired: 4 in, 1 out]
              n339 = Unbundle By Name(w906) -> ("source"=w905:string)
              n340 = Unbundle By Name(w903) -> ("source"=w902:string)
              n341 = Select(t=w902, s=w903, f="DONE") -> (s? t:f=w901:string)
              n342 = Select(t=w905, s=w906, f=w901) -> (s? t:f=w904:string)
            }
            frame "MEMBUFS", "NBUFS", "NMEMBUFS" {
              n343 = Scan From String(format string="%s", input string=w919) -> (output 1=w917:string)  [unwired: 2 in, 4 out]
              n344 = To Lower Case(string=w917) -> (all lower case string=w914:string)
              n345 = Concatenate Strings("set_mbufs " ("key"), w914) -> (w915:string)
              n346 = call "GFITS_toFits.vi"("ms timeout (-1)"=4000, "response Q"="API2GFITS", "key"=w915, "error in (no error)"=w929, "command"="writekey") -> ("error out"=w926:errorcluster, "response"=w923:errorcluster)  [unwired: 4 in, 1 out]
              n347 = Unbundle By Name(w926) -> ("source"=w925:string)
              n348 = Unbundle By Name(w923) -> ("source"=w922:string)
              n349 = Select(t=w922, s=w923, f="DONE") -> (s? t:f=w921:string)
              n350 = Select(t=w925, s=w926, f=w921) -> (s? t:f=w924:string)
            }
            frame "COMPRESS", "COMPRESSION" {
              n351 = call <vilib>:"Trim Whitespace.vi"("string"=w932) -> ("trimmed string"=w931:string)  [unwired: 1 in]
              n352 = Concatenate Strings("set_compress " ("key"), w931) -> (w933:string)
              n353 = call "GFITS_toFits.vi"("ms timeout (-1)"=4000, "response Q"="API2GFITS", "key"=w933, "error in (no error)"=w944, "command"="writekey") -> ("error out"=w941:errorcluster, "response"=w938:errorcluster)  [unwired: 4 in, 1 out]
              n354 = Unbundle By Name(w941) -> ("source"=w940:string)
              n355 = Unbundle By Name(w938) -> ("source"=w937:string)
              n356 = Select(t=w937, s=w938, f="DONE") -> (s? t:f=w936:string)
              n357 = Select(t=w940, s=w941, f=w936) -> (s? t:f=w939:string)
            }
            frame "SHMEM" {
              n358 = Scan From String(format string="%s", input string=w952) -> (output 1=w950:string)  [unwired: 2 in, 4 out]
              n359 = To Lower Case(string=w950) -> (all lower case string=w949:string)
              n360 = case shown="\"on\", \"true\", \"yes\"" w949 {
                tunnel: ["no" "yes"] -> w947
                frame Default {
                }
                frame "on", "true", "yes" {
                }
              }
              n361 = Concatenate Strings("set_shmem " ("key"), w947) -> (w946:string)
              n362 = call "GFITS_toFits.vi"("ms timeout (-1)"=4000, "response Q"="API2GFITS", "key"=w946, "error in (no error)"=w962, "command"="writekey") -> ("error out"=w959:errorcluster, "response"=w956:errorcluster)  [unwired: 4 in, 1 out]
              n363 = Unbundle By Name(w959) -> ("source"=w958:string)
              n364 = Unbundle By Name(w956) -> ("source"=w955:string)
              n365 = Select(t=w955, s=w956, f="DONE") -> (s? t:f=w954:string)
              n366 = Select(t=w958, s=w959, f=w954) -> (s? t:f=w957:string)
            }
            frame "QHDRS", "QUICKHDRS", "QUICKHEADERS" {
              n367 = Scan From String(format string="%s", input string=w971) -> (output 1=w969:string)  [unwired: 2 in, 4 out]
              n368 = To Lower Case(string=w969) -> (all lower case string=w966:string)
              n369 = Concatenate Strings("quickhdrs " ("key"), w966) -> (w967:string)
              n370 = call "GFITS_toFits.vi"("ms timeout (-1)"=4000, "response Q"="API2GFITS", "key"=w967, "error in (no error)"=w981, "command"="writekey") -> ("error out"=w978:errorcluster, "response"=w975:errorcluster)  [unwired: 4 in, 1 out]
              n371 = Unbundle By Name(w978) -> ("source"=w977:string)
              n372 = Unbundle By Name(w975) -> ("source"=w974:string)
              n373 = Select(t=w974, s=w975, f="DONE") -> (s? t:f=w973:string)
              n374 = Select(t=w977, s=w978, f=w973) -> (s? t:f=w976:string)
            }
            frame "ASYNC", "ASYNCMSG", "ASYNCMSGS" {
              n375 = Scan From String(format string="%s", input string=w988) -> (output 1=w986:string)  [unwired: 2 in, 4 out]
              n376 = To Lower Case(string=w986) -> (all lower case string=w983:string)
              n377 = Concatenate Strings("set_async " ("key"), w983) -> (w984:string)
              n378 = call "GFITS_toFits.vi"("ms timeout (-1)"=4000, "response Q"="API2GFITS", "key"=w984, "error in (no error)"=w998, "command"="writekey") -> ("error out"=w995:errorcluster, "response"=w992:errorcluster)  [unwired: 4 in, 1 out]
              n379 = Unbundle By Name(w995) -> ("source"=w994:string)
              n380 = Unbundle By Name(w992) -> ("source"=w991:string)
              n381 = Select(t=w991, s=w992, f="DONE") -> (s? t:f=w990:string)
              n382 = Select(t=w994, s=w995, f=w990) -> (s? t:f=w993:string)
            }
            frame "WRITEHEADER", "WRITEHEADERS" {
              n383 = Scan From String(format string="%s", input string=w1005) -> (output 1=w1003:string)  [unwired: 2 in, 4 out]
              n384 = To Lower Case(string=w1003) -> (all lower case string=w1000:string)
              n385 = Concatenate Strings("set_writeheaders " ("key"), w1000) -> (w1001:string)
              n386 = call "GFITS_toFits.vi"("ms timeout (-1)"=4000, "response Q"="API2GFITS", "key"=w1001, "error in (no error)"=w1015, "command"="writekey") -> ("error out"=w1012:errorcluster, "response"=w1009:errorcluster)  [unwired: 4 in, 1 out]
              n387 = Unbundle By Name(w1012) -> ("source"=w1011:string)
              n388 = Unbundle By Name(w1009) -> ("source"=w1008:string)
              n389 = Select(t=w1008, s=w1009, f="DONE") -> (s? t:f=w1007:string)
              n390 = Select(t=w1011, s=w1012, f=w1007) -> (s? t:f=w1010:string)
            }
            frame "FILEMESSAGE", "FILEMSG" {
              n391 = Scan From String(format string="%s", input string=w1021) -> (output 1=w1017:string)  [unwired: 2 in, 4 out]
              n392 = Concatenate Strings("set_filemsg " ("key"), w1017) -> (w1018:string)
              n393 = call "GFITS_toFits.vi"("ms timeout (-1)"=4000, "response Q"="API2GFITS", "key"=w1018, "error in (no error)"=w1031, "command"="writekey") -> ("error out"=w1028:errorcluster, "response"=w1025:errorcluster)  [unwired: 4 in, 1 out]
              n394 = Unbundle By Name(w1028) -> ("source"=w1027:string)
              n395 = Unbundle By Name(w1025) -> ("source"=w1024:string)
              n396 = Select(t=w1024, s=w1025, f="DONE") -> (s? t:f=w1023:string)
              n397 = Select(t=w1027, s=w1028, f=w1023) -> (s? t:f=w1026:string)
            }
            frame "DATACUBE", "NZIM", "NZIMAGES", "ZAXIS", "ZIMAGES" {
              n398 = Scan From String(format string="%s", input string=w1038) -> (output 1=w1036:string)  [unwired: 2 in, 4 out]
              n399 = To Lower Case(string=w1036) -> (all lower case string=w1033:string)
              n400 = Concatenate Strings("nz " ("key"), w1033) -> (w1034:string)
              n401 = call "GFITS_toFits.vi"("ms timeout (-1)"=4000, "response Q"="API2GFITS", "key"=w1034, "error in (no error)"=w1048, "command"="writekey") -> ("error out"=w1045:errorcluster, "response"=w1042:errorcluster)  [unwired: 4 in, 1 out]
              n402 = Unbundle By Name(w1045) -> ("source"=w1044:string)
              n403 = Unbundle By Name(w1042) -> ("source"=w1041:string)
              n404 = Select(t=w1041, s=w1042, f="DONE") -> (s? t:f=w1040:string)
              n405 = Select(t=w1044, s=w1045, f=w1040) -> (s? t:f=w1043:string)
            }
            frame "IMAGENUMFORMAT", "IMNUMFORMAT", "NUMFORMAT" {
              n406 = Scan From String(format string="%s", input string=w1057) -> (output 1=w1055:string)  [unwired: 2 in, 4 out]
              n407 = To Lower Case(string=w1055) -> (all lower case string=w1052:string)
              n408 = Concatenate Strings("set_imnumformat " ("key"), w1052) -> (w1053:string)
              n409 = call "GFITS_toFits.vi"("ms timeout (-1)"=5000, "response Q"="API2GFITS", "key"=w1053, "error in (no error)"=w1060, "command"="writekey") -> ("error out"=w1051:errorcluster)  [unwired: 4 in, 2 out]
              n410 = Unbundle By Name(w1051) -> ("source"=w1050:string)
            }
            frame "HDR", "HDRVAR", "HDR_VAR", "VAR" {
              n411 = call "CMN_Str2Arr.vi"("separator"=",", "string in"=w1064) -> ("Array out"=w1062:string[])  [unwired: 2 in, 7 out]
              n412 = for {
                tunnel: [w1075] -> w1067
                tunnel: w1066 -> [w1074]
                tunnel: [w1072] -> w1065
                tunnel: w1062 -> [w1069] mode=indexing
                n413 = call <vilib>:"Trim Whitespace.vi"("string"=w1069) -> ("trimmed string"=w1070:string)  [unwired: 1 in]
                n414 = call "GFITS_toFits.vi"("ms timeout (-1)"=5000, "response Q"="API2GFITS", "key"=w1070, "error in (no error)"=w1074, "command"="writekey" ("string")) -> ("response"=w1072:errorcluster)  [unwired: 4 in, 2 out]
                n415 = Unbundle By Name(w1072) -> ("source"=w1079:string)
                n416 = Unbundle By Name(w1072) -> ("source"=w1078:string)
                n417 = Select(t=w1078, s=w1072, f="DONE") -> (s? t:f=w1077:string)
                n418 = Select(t=w1079, s=w1072, f=w1077) -> (s? t:f=w1075:string)
              }
            }
            frame "HDRPREALLOC", "KEYPREALLOC" {
              n419 = Scan From String(format string="%s" ("Format String"), input string=w1087) -> (output 1=w1085:string)  [unwired: 2 in, 4 out]
              n420 = To Lower Case(string=w1085) -> (all lower case string=w1088:string)
              n421 = case shown="Default" w1088 {
                tunnel: [w1098 -1 ("nkeys in")] -> w1081
                tunnel: w1085 -> [w1101 _]
                tunnel: w1084 -> [_ w1103]
                tunnel: [w1097 w1103] -> w1083
                frame Default {
                  n422 = Scan From String(format string="%d", input string=w1101) -> (error out=w1097:errorcluster, output 1=w1100:i32)  [unwired: 2 in, 3 out]
                  n423 = Select(t=-1, s=w1097, f=w1100) -> (s? t:f=w1098:i32)
                }
                frame "", "auto", "dynamic" {
                }
              }
              n424 = case shown="No Error" w1083 {
                selector: w1083 -> [w1091 w1096]
                tunnel: [w1091 w1094] -> w1082
                tunnel: w1081 -> [w1090 _]
                tunnel: ["DONE" ("f") w1093] -> w1080
                frame No Error {
                  n425 = call "GFITS_VAR_preallocHdrs.vi"("nkeys in"=w1090, "action"=enum16{"read", "write"}."write") -> ()  [unwired: 14 out]
                }
                frame Error {
                  w1093 = "ERROR \"auto\" or <number>" ("f")
                  n426 = Bundle By Name(cluster=w1096, "code"=-22, "source"=w1093) -> (w1094:errorcluster)
                }
              }
            }
            frame "HDRMODE", "KEYMODE" {
              n427 = Scan From String(format string="%s" ("Format String"), input string=w1112) -> (output 1=w1110:string)  [unwired: 2 in, 4 out]
              n428 = To Lower Case(string=w1110) -> (all lower case string=w1113:string)
              n429 = case shown="\"\", \"auto\", \"dynamic\"" w1113 {
                tunnel: w1110 -> [_ _ _]
                tunnel: w1109 -> [w1123 w1125 w1129]
                tunnel: [w1123 w1125 w1128] -> w1108
                tunnel: [FALSE ("nkeys in") TRUE ("nkeys in") FALSE ("nkeys in")] -> w1105
                frame "", "auto", "dynamic" {
                }
                frame "static" {
                }
                frame Default {
                  n430 = Bundle By Name(cluster=w1129, "status"=TRUE) -> (w1128:errorcluster)
                }
              }
              n431 = case shown="No Error" w1108 {
                selector: w1108 -> [w1117 w1121]
                tunnel: [w1117 w1119] -> w1107
                tunnel: ["DONE" ("f") w1118] -> w1106
                tunnel: w1105 -> [w1114 _]
                frame No Error {
                  n432 = call "GFITS_VAR_staticHdrs.vi"("static in"=w1114, "action"=enum16{"read", "write"}."write") -> ()  [unwired: 14 out]
                }
                frame Error {
                  w1118 = "ERROR <dynamic | static>" ("f")
                  n433 = Bundle By Name(cluster=w1121, "code"=-22, "source"=w1118) -> (w1119:errorcluster)
                }
              }
            }
            frame "TESTMODE", "TMPMODE" {
              n434 = Scan From String(format string="%s" ("Format String"), input string=w1138) -> (remaining string=w1130:string, output 1=w1136:string)  [unwired: 2 in, 3 out]
              n435 = To Lower Case(string=w1136) -> (all lower case string=w1135:string)
              n436 = case shown="\"0\", \"disable\", \"false\", \"no\", \"off\"" w1135 {
                tunnel: [w1139 "DONE" ("f") "DONE" ("f")] -> w1134
                tunnel: w1133 -> [w1143 w1155 w1171]
                tunnel: [w1142 w1155 w1171] -> w1132
                tunnel: w1131 -> [_ w1148 w1170]
                tunnel: w1130 -> [_ _ w1161]
                frame Default {
                  w1139 = "Bad argument <on | off>" ("source")
                  n437 = Bundle By Name(cluster=w1143, "status"=TRUE, "code"=-22, "source"=w1139) -> (w1142:errorcluster)
                }
                frame "1", "enable", "on", "true", "yes" {
                  w1150 = TRUE
                  w1147 = "autonumbering" ("name")
                  n438 = call-poly "DatabaseHand_Get.vi"("default value"=TRUE, "name"=w1147, "Database RefNum in"=w1148) -> ("value"=→"origautonum":bool, "Database RefNum out"=w1145:T2)  [unwired: 2 in, 5 out]
                  n439 = call-poly "DatabaseHand_Set.vi"("name"=w1147, "value"=FALSE, "Database RefNum in"=w1145) -> ("Database RefNum out"=w1154:T2)  [unwired: 5 in, 3 out]
                  n440 = call-poly "DatabaseHand_Set.vi"("name"="fitsoverride", "value"=w1150, "Database RefNum in"=w1154) -> ("Database RefNum out"=w1152:T2)  [unwired: 5 in, 3 out]
                  n441 = call-poly "DatabaseHand_Set.vi"("name"="usetestdir", "value"=w1150, "Database RefNum in"=w1152) -> ()  [unwired: 5 in, 4 out]
                }
                frame "0", "disable", "false", "no", "off" {
                  w1164 = FALSE
                  n442 = local read "origautonum"() -> (w1162:bool)
                  n443 = call-poly "DatabaseHand_Set.vi"("name"="autonumbering", "value"=w1162, "Database RefNum in"=w1170) -> ("Database RefNum out"=w1168:T2)  [unwired: 5 in, 3 out]
                  n444 = Scan From String(format string="%s", input string=w1161) -> (output 1=w1159:string)  [unwired: 2 in, 4 out]
                  n445 = To Lower Case(string=w1159) -> (all lower case string=w1158:string)
                  n446 = case shown="\"noinc\"" w1158 {
                    tunnel: [TRUE FALSE] -> w1157
                    frame Default {
                    }
                    frame "noinc" {
                    }
                  }
                  n447 = call-poly "DatabaseHand_Set.vi"("name"="fitsoverride", "value"=w1164, "Database RefNum in"=w1168) -> ("Database RefNum out"=w1166:T2)  [unwired: 5 in, 3 out]
                  n448 = call-poly "DatabaseHand_Set.vi"("name"="usetestdir", "value"=w1164, "Database RefNum in"=w1166) -> ("Database RefNum out"=w1163:T2)  [unwired: 5 in, 3 out]
                  n449 = call "GFITS_buildNextImageName.vi"("incnumber"=w1157, "Database RefNum"=w1163) -> ()  [unwired: 2 in, 6 out]
                }
              }
            }
            frame "GEOMHDRMODE" {
              n450 = Scan From String(format string="%s" ("Format String"), input string=w1182) -> (output 1=w1180:string)  [unwired: 2 in, 4 out]
              n451 = To Lower Case(string=w1180) -> (all lower case string=w1183:string)
              n452 = case shown="\"static\"" w1183 {
                tunnel: w1180 -> [_ _ _]
                tunnel: w1179 -> [w1193 w1195 w1199]
                tunnel: [w1193 w1195 w1198] -> w1178
                tunnel: [FALSE ("nkeys in") TRUE ("nkeys in") FALSE ("nkeys in")] -> w1175
                frame "", "auto", "dynamic" {
                }
                frame "static" {
                }
                frame Default {
                  n453 = Bundle By Name(cluster=w1199, "status"=TRUE) -> (w1198:errorcluster)
                }
              }
              n454 = case shown="No Error" w1178 {
                selector: w1178 -> [w1187 w1191]
                tunnel: [w1187 w1189] -> w1177
                tunnel: ["DONE" ("f") w1188] -> w1176
                tunnel: w1175 -> [w1184 _]
                frame No Error {
                  n455 = call "GFITS_VAR_fstaticGeomHdrs.vi"("static in"=w1184, "action"=enum16{"read", "write"}."write") -> ()  [unwired: 14 out]
                }
                frame Error {
                  w1188 = "ERROR <dynamic | static>" ("f")
                  n456 = Bundle By Name(cluster=w1191, "code"=-22, "source"=w1188) -> (w1189:errorcluster)
                }
              }
            }
            frame "ROI" {
              n457 = Scan From String(format string="%s", input string=w1204) -> (output 1=w1202:string)  [unwired: 2 in, 4 out]
              n458 = To Lower Case(string=w1202) -> (all lower case string=w1201:string)
              n459 = case shown="\"0\", \"disable\", \"false\", \"no\", \"none\", \"off\"" w1201 {
                tunnel: w1204 -> [w1215 _]
                tunnel: [w1208 w1228] -> w1206
                tunnel: [w1207 "DONE" ("f")] -> w1205
                tunnel: w1200 -> [_ w1229]
                frame Default {
                  n460 = Scan From String(format string="%d %d %d %d", input string=w1215) -> (error out=w1213:errorcluster, output 1=w1212:i32, output 2=w1211:i32, output 3=w1210:i32, output 4=w1209:i32)  [unwired: 2 in, 6 out]
                  n461 = case shown="No Error" w1213 {
                    selector: w1213 -> [w1222 w1224]
                    tunnel: w1212 -> [w1220 _]
                    tunnel: w1211 -> [w1219 _]
                    tunnel: w1210 -> [w1218 _]
                    tunnel: w1209 -> [w1217 _]
                    tunnel: [w1221 w1224] -> w1208
                    tunnel: ["DONE" ("f") "usage: <xstart> <ystart> <xlen> <ylen> (all numbers)" ("f")] -> w1207
                    frame No Error {
                      n462 = call "GFITS_LibSetRoi.vi"("ylen"=w1217, "ystart"=w1219, "xlen"=w1218, "xstart"=w1220, "error in (no error)"=w1222) -> ("error IO"=w1221:errorcluster)  [unwired: 6 out]
                    }
                    frame Error {
                    }
                  }
                }
                frame "0", "disable", "false", "no", "none", "off" {
                  w1226 = u32 0 ("xlen")
                  w1227 = u32 0 ("xstart")
                  n463 = call "GFITS_LibSetRoi.vi"("ylen"=w1226, "ystart"=w1227, "xlen"=w1226, "xstart"=w1227, "error in (no error)"=w1229) -> ("error IO"=w1228:errorcluster)  [unwired: 6 out]
                }
              }
            }
          }
          n464 = Unbundle By Name(w500) -> ("source"=w506:string)
        }
        frame "KEY", "KEYWORD" {
          n465 = global read "GFITS_Gbls.vi" "GFITS_Def_Head_timing"() -> (w1237:string)
          n466 = call "CMN_TrimStringWhitespace.vi"("Both Ends?(T)"=TRUE, "string"=w1247) -> ("trimmed string"=w1233:string)  [unwired: 8 out]
          n467 = Scan From String(format string="%s" ("Format String"), input string=w1233) -> (remaining string=w1231:string, output 1=w1244:string)  [unwired: 2 in, 3 out]
          n468 = To Upper Case(1:w1244) -> (0:w1239:string)
          n469 = call "CMN_Str2Arr.vi"("strip quotation marks"=TRUE, "separator"=",", "string in"=w1231) -> ("Array out"=w1234:string[])  [unwired: 1 in, 7 out]
          n470 = for {
            tunnel: [w1256] -> w1242
            tunnel: w1241 -> [w1255]
            tunnel: [w1254] -> w1240
            tunnel: w1239 -> [w1253]
            tunnel: w1238 -> [w1252]
            tunnel: w1237 -> [w1251]
            tunnel: w1236 -> [w1250]
            tunnel: w1234 -> [w1249] mode=indexing
            tunnel: w1232 -> [w1248]
            n471 = case shown="\"GET\"" w1253 {
              selector: w1253 -> [w1257 _ _ _ _]
              tunnel: [w1258 "DONE" ("data string") w1276 w1315 w1357] -> w1256
              tunnel: w1255 -> [w1260 w1266 w1280 w1312 w1359]
              tunnel: [w1259 w1265 w1280 w1311 w1358] -> w1254
              tunnel: w1252 -> [_ w1264 w1272 w1307 w1356]
              tunnel: w1251 -> [_ _ w1275 w1310 _]
              tunnel: w1250 -> [_ _ _ _ _]
              tunnel: w1249 -> [_ w1263 w1269 w1304 w1353]
              tunnel: w1248 -> [_ w1262 w1268 w1303 w1352]
              frame Default {
                n472 = call "CMN_BadParamMsg.vi"("valid params"=string[] ["ADD <name> <dbs [name] || [type] <name> // <comment>", "DELETE <name>", "PREVIEW", "GET <name | ALL | PREVIEW>"], "error in (no error)"=w1260, "parameter"=w1257) -> ("error out"=w1259:errorcluster)  [unwired: 1 in, 7 out]
                n473 = Unbundle By Name(w1259) -> ("source"=w1258:string)
              }
              frame "ADD", "SET" {
                n474 = call "GFITS_AddKeyword.vi"("auxhdr"=w1262, "Database RefNum"=w1264, "error in"=w1266, "command in"=w1263) -> ("error out"=w1265:errorcluster)  [unwired: 7 out]
              }
              frame "DELETE" {
                n475 = call "GFITS_SelectHdrFile.vi"("auxhdr"=w1268, "line in"=w1269, "Database RefNum"=w1272) -> ("path out"=w1271:path, "line out"=w1270:string)  [unwired: 7 out]
                n476 = Scan From String(format string="%s" ("Format String"), input string=w1270) -> (output 1=w1278:string)  [unwired: 2 in, 4 out]
                n477 = To Upper Case(1:w1278) -> (0:w1277:string)
                n478 = call "GFITS_Readfile2fits.vi"("def_timing"=w1275, "file"=w1271) -> ("all keys"=w1274:string[][], "number of total keywords"=w1273:i32)  [unwired: 8 out]
                n479 = case shown="Default" w1277 {
                  selector: w1277 -> [_ w1283]
                  tunnel: w1274 -> [_ w1287]
                  tunnel: w1271 -> [_ w1289]
                  tunnel: w1273 -> [_ w1288]
                  tunnel: ["ERROR nothing to delete" w1282] -> w1276
                  frame "", " " {
                  }
                  frame Default {
                    n480 = Build Array(w1287) -> (w1286:string[][][])
                    n481 = call "GFITS_FindKeywordFromArray.vi"("Keyword"=w1283, "Keywords"=w1286) -> ("found"=w1284:bool, "indexes"=w1285:i16[])  [unwired: 8 out]
                    n482 = case shown="True" w1284 {
                      tunnel: w1289 -> [_ w1300]
                      tunnel: w1288 -> [_ _]
                      tunnel: w1287 -> [_ w1298]
                      tunnel: w1285 -> [_ w1297]
                      tunnel: w1283 -> [w1292 _]
                      tunnel: [w1290 "DONE"] -> w1282
                      frame False {
                        n483 = Concatenate Strings("ERROR keyword " ("data string"), w1292, " NOT FOUND" ("string")) -> (w1290:string)
                      }
                      frame True {
                        n484 = Index Array(array=w1297, index=0 ("Index")) -> (element=w1295:i16)
                        n485 = Delete From Array(array=w1298, index (row)=w1295) -> (array with subset deleted=w1299:string[][])  [unwired: 2 in, 1 out]
                        n486 = call "GFITS_Fits2File.vi"("write to file?"=TRUE, "Keywords"=w1299, "append to file? (new file:F)"=FALSE, "filename"=w1300) -> ()  [unwired: 1 in, 7 out]
                      }
                    }
                  }
                }
              }
              frame "GET" {
                n487 = call "GFITS_SelectHdrFile.vi"("auxhdr"=w1303, "line in"=w1304, "Database RefNum"=w1307) -> ("path out"=w1306:path, "line out"=w1305:string)  [unwired: 7 out]
                n488 = Scan From String(format string="%s" ("Format String"), input string=w1305) -> (remaining string=w1308:string, output 1=w1314:string)  [unwired: 2 in, 3 out]
                n489 = To Upper Case(1:w1314) -> (0:w1313:string)
                n490 = call "GFITS_Readfile2fits.vi"("def_timing"=w1310, "file"=w1306) -> ("all keys"=w1309:string[][])  [unwired: 9 out]
                n491 = case shown="\"PREVIEW\"" w1313 {
                  selector: w1313 -> [_ w1322 _ _]
                  tunnel: w1309 -> [_ w1331 w1342 _]
                  tunnel: w1306 -> [_ _ w1341 w1347]
                  tunnel: [w1318 w1325 w1338 w1348] -> w1315
                  tunnel: w1312 -> [w1321 w1323 w1340 w1350]
                  tunnel: [w1320 w1323 w1339 w1349] -> w1311
                  tunnel: w1307 -> [_ _ _ w1346]
                  tunnel: w1308 -> [_ _ _ w1345]
                  frame "", " " {
                    w1318 = " nothing to get"
                    n492 = Bundle By Name(cluster=w1321, "source"=w1318, "code"=-22, "status"=FALSE) -> (w1320:errorcluster)
                  }
                  frame Default {
                    w1329 = 0 ("Index")
                    n493 = Build Array(w1331) -> (w1330:string[][][])
                    n494 = call "GFITS_FindKeywordFromArray.vi"("Keyword"=w1322, "Keywords"=w1330) -> ("values"=w1327:string[][], "indexes"=w1328:i16[])  [unwired: 8 out]
                    n495 = Index Array(array=w1328, index=w1329) -> (element=w1326:i16)
                    n496 = Index Array(array=w1327, index (row)=w1329) -> (element=w1324:string[])  [unwired: 1 in]
                    n497 = case shown="-1" w1326 {
                      tunnel: [w1332 w1336] -> w1325
                      tunnel: w1324 -> [_ w1337]
                      tunnel: w1322 -> [w1334 _]
                      frame -1 {
                        n498 = Concatenate Strings("ERROR keyword " ("string"), w1334, " NOT FOUND") -> (w1332:string)
                      }
                      frame Default {
                        n499 = call "CMN_Arr2Str.vi"("Array in"=w1337) -> ("string out"=w1336:string)  [unwired: 10 out]
                      }
                    }
                  }
                  frame "ALL" {
                    n500 = call "GFITS_Fits2File.vi"("write to file?"=FALSE, "error in (no error)"=w1340, "Keywords"=w1342, "filename"=w1341) -> ("error out"=w1339:errorcluster, "string out"=w1338:string)  [unwired: 1 in, 5 out]
                  }
                  frame "PREVIEW" {
                    n501 = call "GFITS_KeyPreview.vi"("nd queue"=TRUE, "template path"=w1347, "error in (no error)"=w1350, "args"=w1345, "Database RefNum in"=w1346) -> ("error out"=w1349:errorcluster, "preview"=w1348:string)  [unwired: 5 out]
                  }
                }
              }
              frame "PREVIEW" {
                n502 = call "GFITS_SelectHdrFile.vi"("auxhdr"=w1352, "line in"=w1353, "Database RefNum"=w1356) -> ("path out"=w1354:path, "line out"=w1355:string)  [unwired: 7 out]
                n503 = call "GFITS_KeyPreview.vi"("nd queue"=TRUE, "template path"=w1354, "error in (no error)"=w1359, "args"=w1355, "Database RefNum in"=w1356) -> ("error out"=w1358:errorcluster, "preview"=w1357:string)  [unwired: 5 out]
              }
            }
          }
          n504 = Unbundle By Name(w1240) -> ("source"=w1245:string)
        }
        frame "VERSION" {
          n505 = Search 1D Array(1D array=w1364, element="-full") -> (index of element=w1362:i32)  [unwired: 1 out]
          n506 = Greater Or Equal To 0?(x=w1362) -> (x >= 0?=w1361:bool)
          n507 = property on="caller path" class="Path"() -> ("Value"=w1360:path)  [unwired: 2 in, 2 out]
          n508 = call "CMN_modinfo.vi"("error in (no error)"=w1366, "full"=w1361, "caller path"=w1360) -> ("error out"=w1365:errorcluster, "INFO"=w1367:string)  [unwired: 7 out]
        }
        frame "IMLIST", "IMLOG" {
          w1375 = "GFITSAPI2IMLOGQ" ("responseQ")
          n509 = call <vilib>:"Trim Whitespace.vi"("string"=w1369) -> ("trimmed string"=w1368:string)  [unwired: 1 in]
          n510 = Bundle By Name(cluster="cmd struct", "command"=w1368, "responseQ"=w1375) -> (w1379:T1)
          n511 = Obtain Queue(name (unnamed)="GFITS_IMLOGQ", element data type="cmd struct") -> (queue out=w1378:refnum<queue>)  [unwired: 3 in, 2 out]
          n512 = Enqueue Element(queue=w1378, element=w1379) -> (queue out=w1377:refnum<queue>, error out=w1376:errorcluster)  [unwired: 1 in, 2 out]
          n513 = Obtain Queue(name (unnamed)=w1375, element data type=w1375) -> (queue out=w1374:refnum<queue>)  [unwired: 3 in, 2 out]
          n514 = Dequeue Element(queue=w1374, timeout in ms (-1)=5000, error in (no error)=w1376) -> (queue out=w1372:refnum<queue>, element=w1371:string)  [unwired: 2 out]
          n515 = Release Queue(queue=w1377) -> ()  [unwired: 1 in, 4 out]
          n516 = Release Queue(queue=w1372) -> ()  [unwired: 1 in, 4 out]
        }
        frame "", "?", "help" {
          n517 = call "CMN_BadParamMsg.vi"("valid params"=string[] ["GET <..>", "SET <..>", "KEY <..>", "VERSION", "LOCK", "WRITEBUF"], "error in (no error)"=w1385, "parameter"=w1386) -> ("error out"=w1384:errorcluster)  [unwired: 1 in, 7 out]
          n518 = Unbundle By Name(w1384) -> ("source"=w1383:string)
        }
      }
      n519 = Current VI's Path() -> (path=w26:path)
      n520 = Strip Path(path=w26) -> (name=w25:string)  [unwired: 1 out]
      n521 = Concatenate Strings("ERROR ", w25, " " ("string"), w13) -> (w24:string)
      n522 = Select(t=w24, s=w23, f=w21) -> (s? t:f=w22:string)
    }
    frame True {
    }
  }
  "error out" <- w1
  "ImmedReplyString" <- w5
